vi "STD Cal Data.vi"(8 "error in":errorcluster caption="에러 입력(에러 없음)", 9 "Data in":string[][](array[string]), 10 "문자열":string, 11 "Func_ext":string) -> (0 "error out":errorcluster caption="에러 출력", 1 "Data Out":string[][](array[string]), 3 "Func_ext Out":string, 4 "Data Out 2":string[](array[string]), 6 "Cal STD":string[][](array[string]))   [LabVIEW 2020]
uses:
  Controls/Cmd_Var Data IO.ctl
  Controls/Cmd_File path.ctl
  Controls/Cmd_File Type.ctl
  Controls/Cmd_STD select.ctl
  <vilib>/Utility/file.llb/Read Delimited Spreadsheet (string).vi
  Public/Polymorph/Data Class_2D Str.vi
  Public/Polymorph/Array Dedup_1D Str.vi
  Public/Polymorph/Sort_2D Str.vi
  Variables/Global_Cal Info.vi
panel:
  out "Cal STD in":string[][](array[string])
  out "Condition Default":string[][](array[string])
  out "데이터오류?":bool
  out "생성오류?":bool
  out "Condition":string[][](array[string])
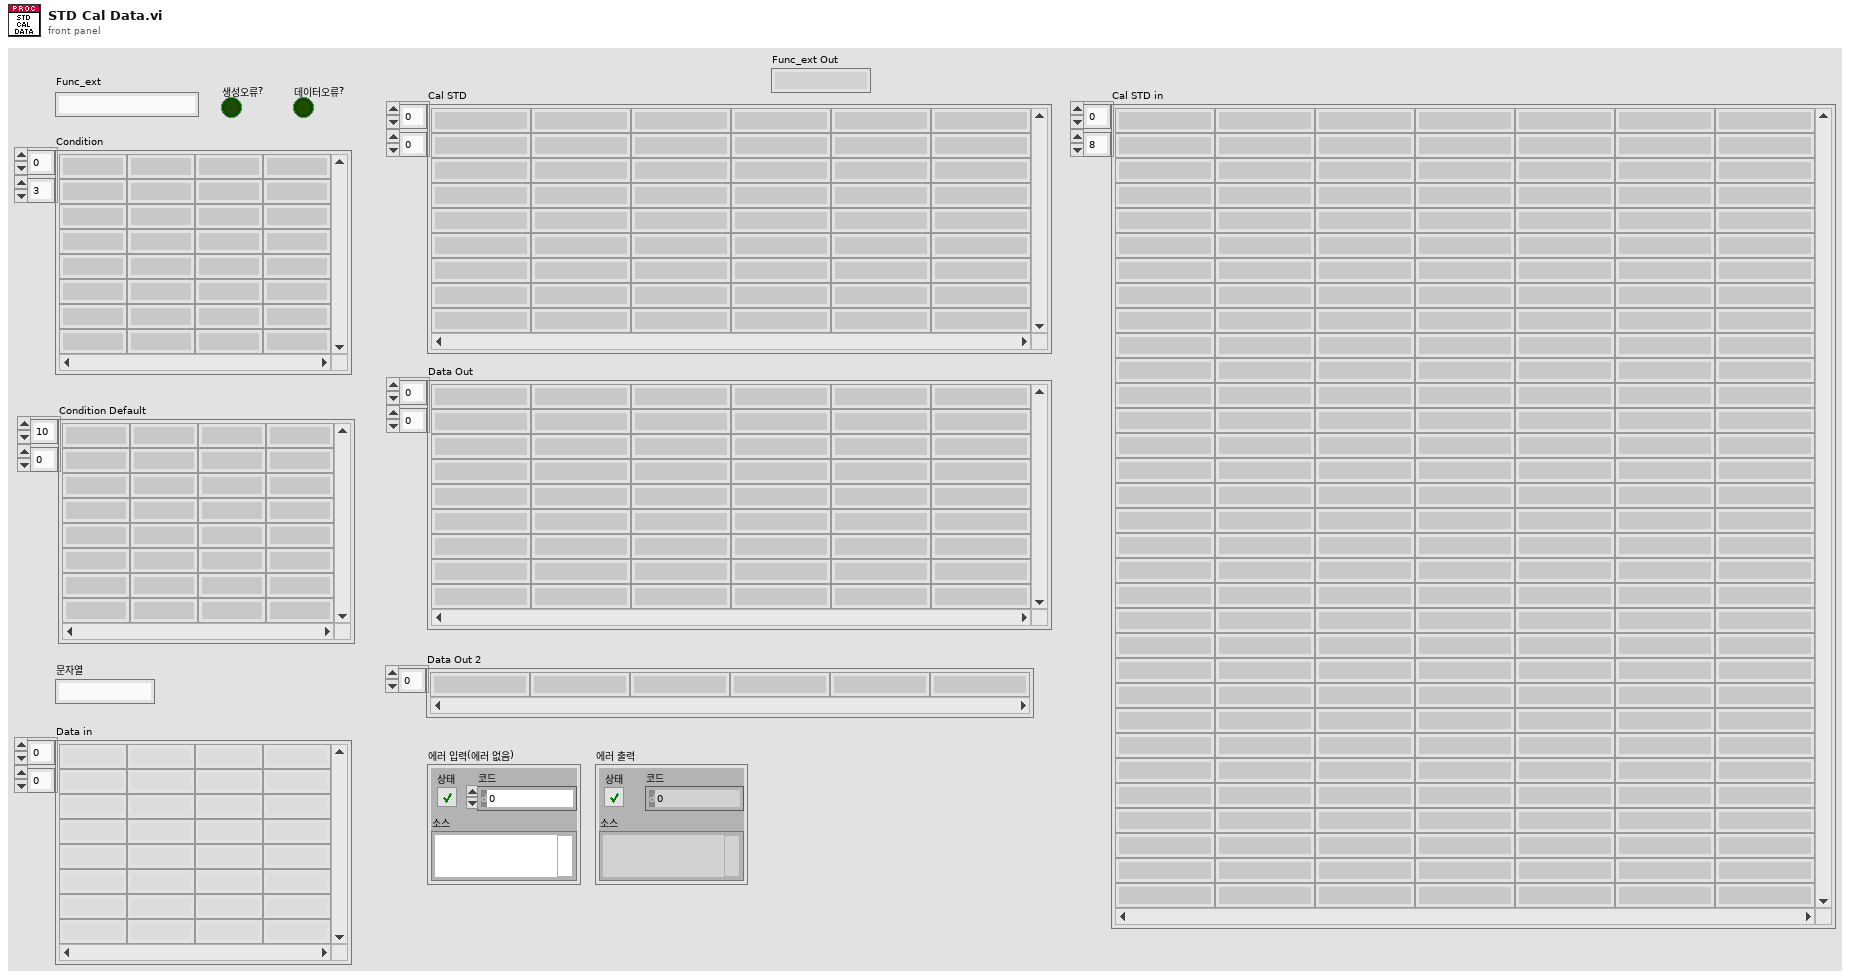
[diagram p1: front panel]
types:
  T1 = typedef "Cmd_Var Data IO.ctl" = enum16{"Condition", "Condition Default", "Condition_Temp", "Resolution", "Resolution Default", "Resolution Old", "Spec", "Spec Default", "Spec Old", "Spec Temp", "Result", "Result2", "Result3", "Result_Temp", "Result_ADJ", "Result_ADJ2", "STD1", "STD2", "STD3", "STD4", "STD5", "STD Temp", "CMC", "CMC Default"}
  T2 = typedef "Cmd_File Type.ctl" = enum16{"엑셀", "엑셀(2003)", "텍스트", "설정", "2진", "VI", "CSV", "LOG", "폴더"}
  T3 = typedef "Cmd_File path.ctl" = enum16{"에러로그", "데이터파일경로", "성적서원본", "지난성적서", "Data Files", "경로생성", "Updater", "Template", "설정파일경로", "FTP Upload", "Update 경로", "어플리케이션"}
  T4 = typedef "Cmd_STD select.ctl" = enum16{"기본", "DMM", "Electronic Micrometer", "Fine Angle Generator", "Measuring Projector", "Precision Square", "Power Supply", "Ring Gauge", "Straight Edge", "Thermo-Hygrometer", "Calibrator"}
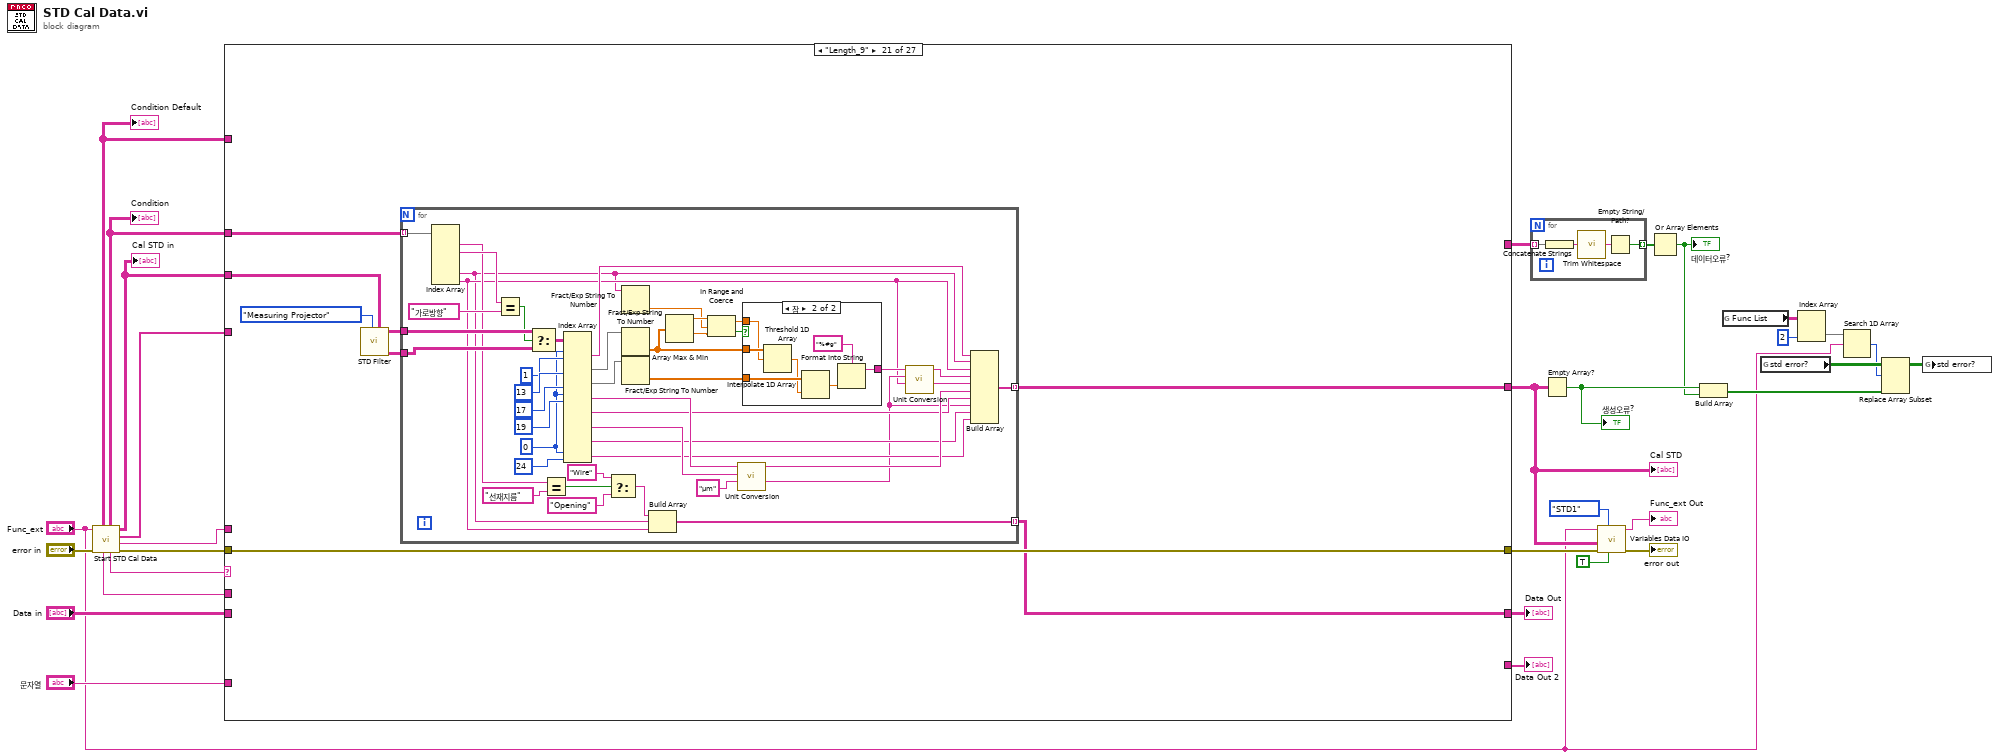
[diagram p0: block diagram]
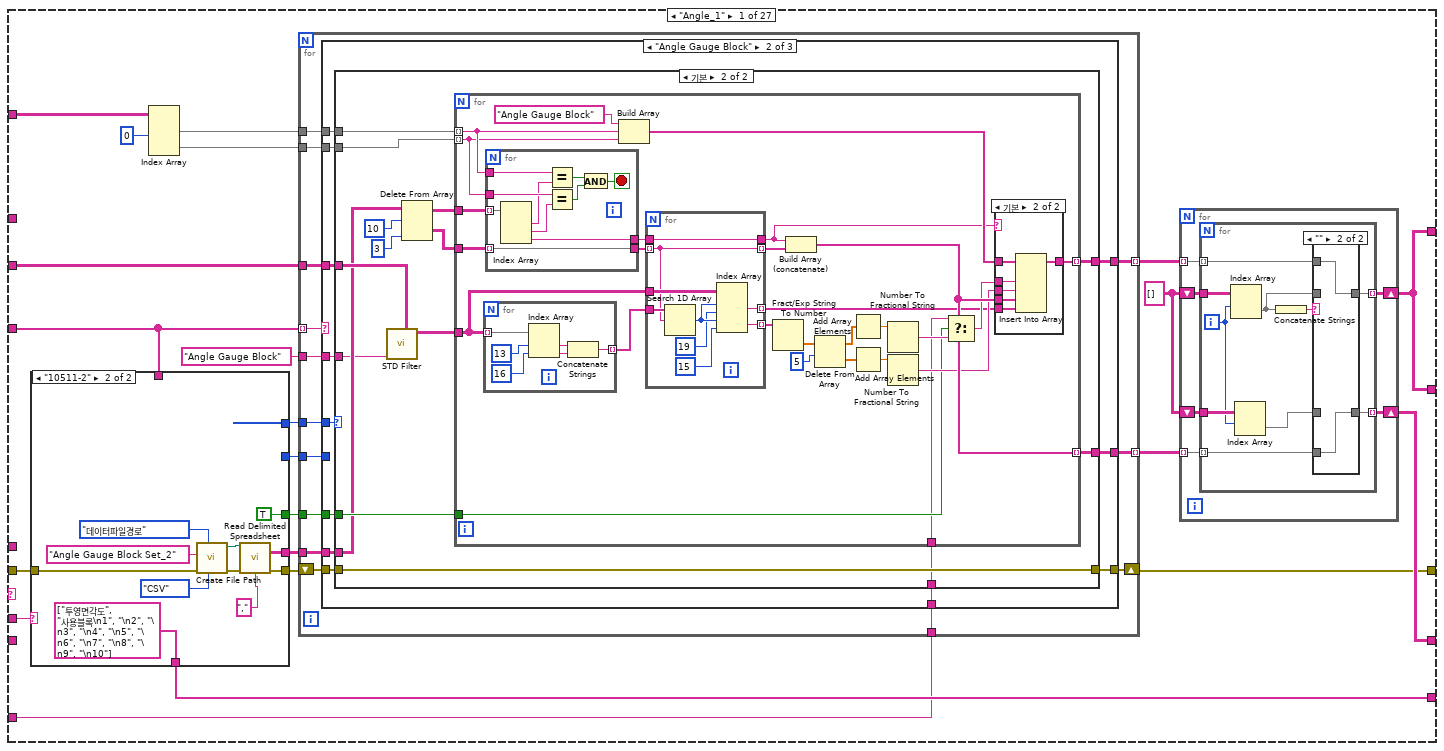
[diagram p2: hidden frame]
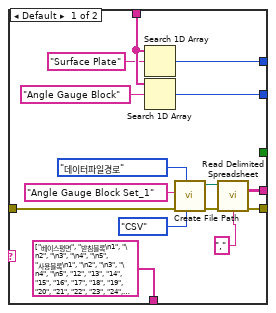
[diagram p3: hidden frame]
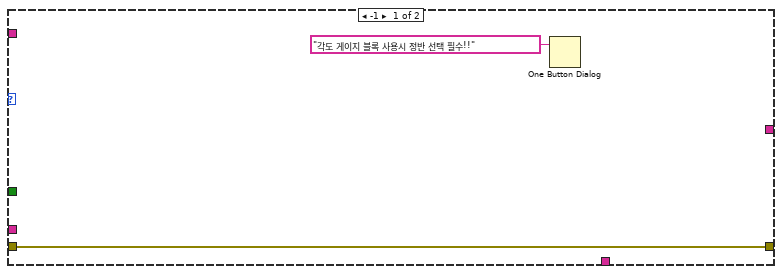
[diagram p6: hidden frame]
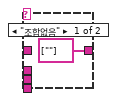
[diagram p7: hidden frame]
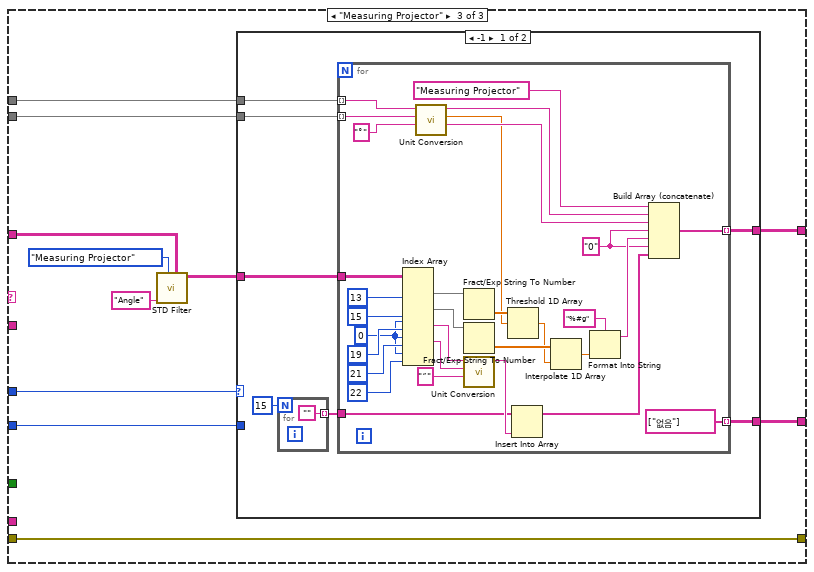
[diagram p8: hidden frame]
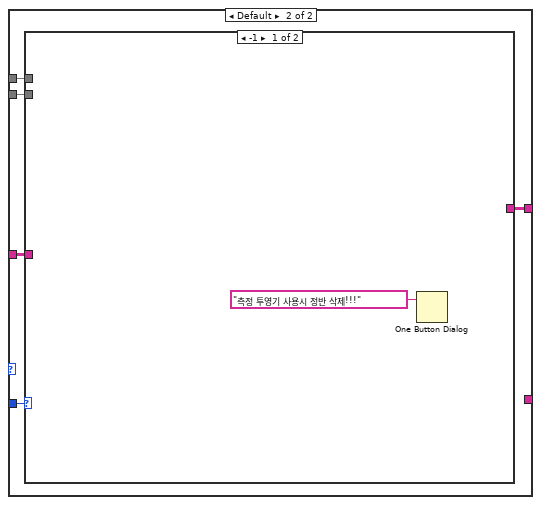
[diagram p9: hidden frame]
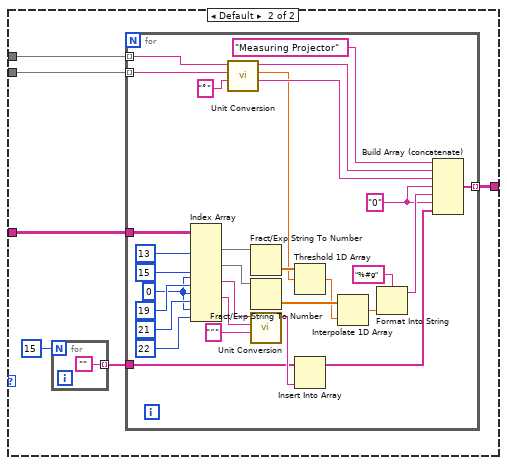
[diagram p10: hidden frame]
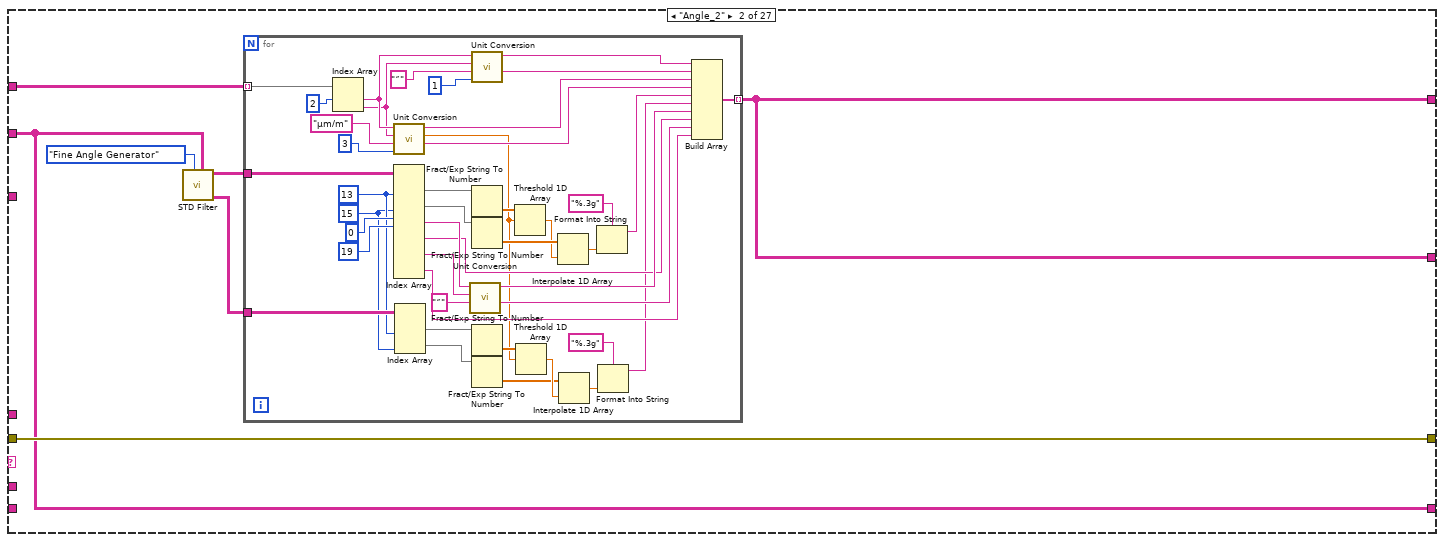
[diagram p11: hidden frame]
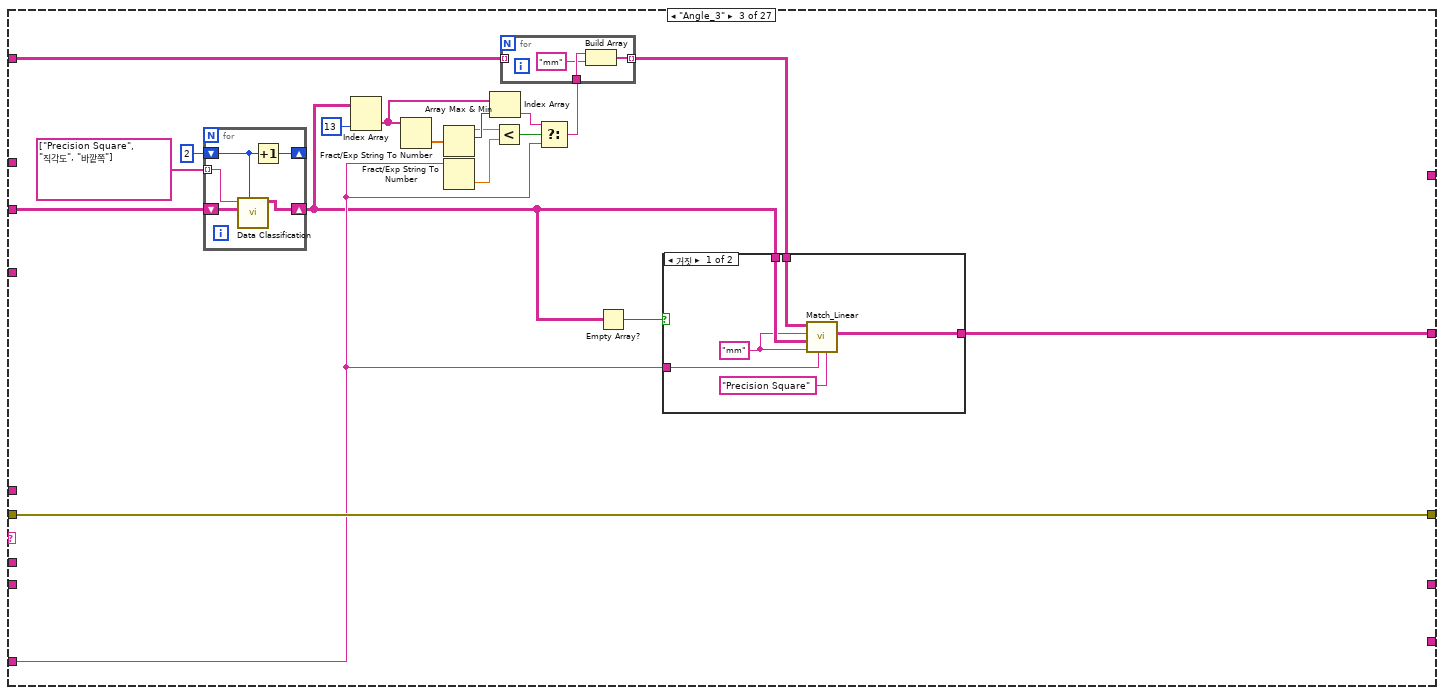
[diagram p12: hidden frame]
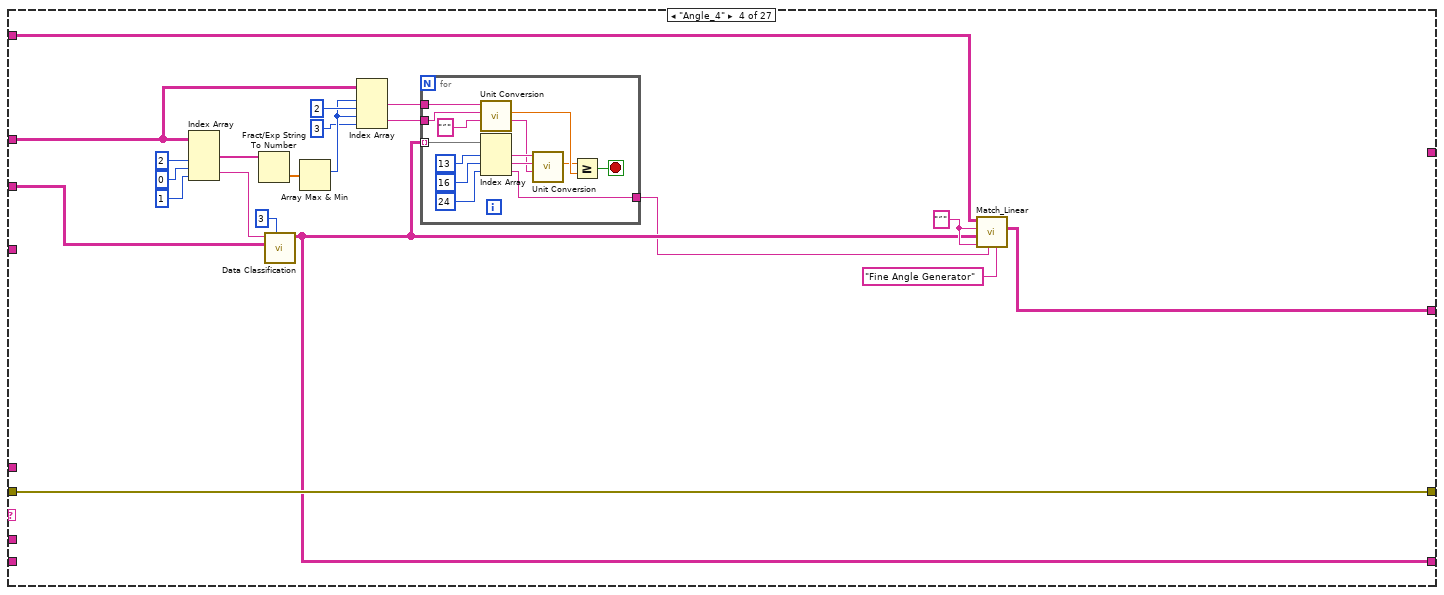
[diagram p14: hidden frame]
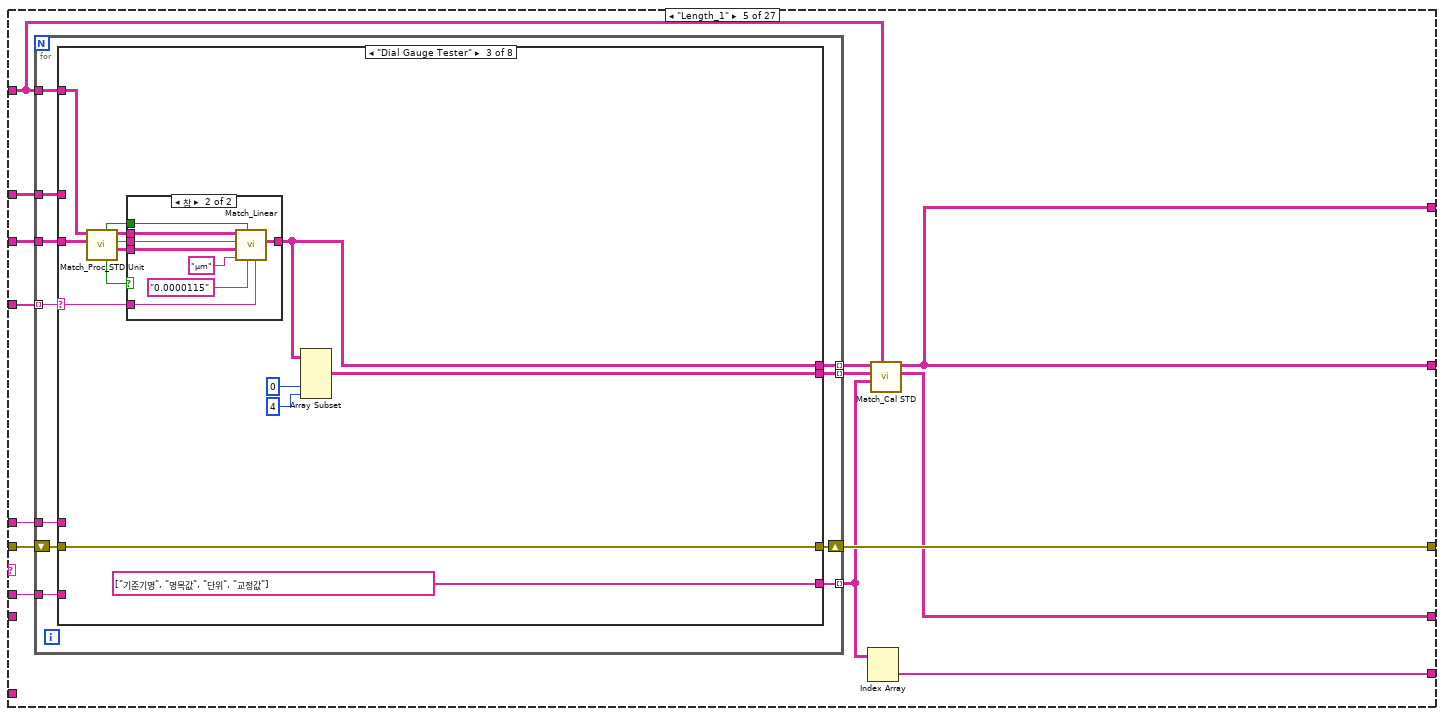
[diagram p15: hidden frame]
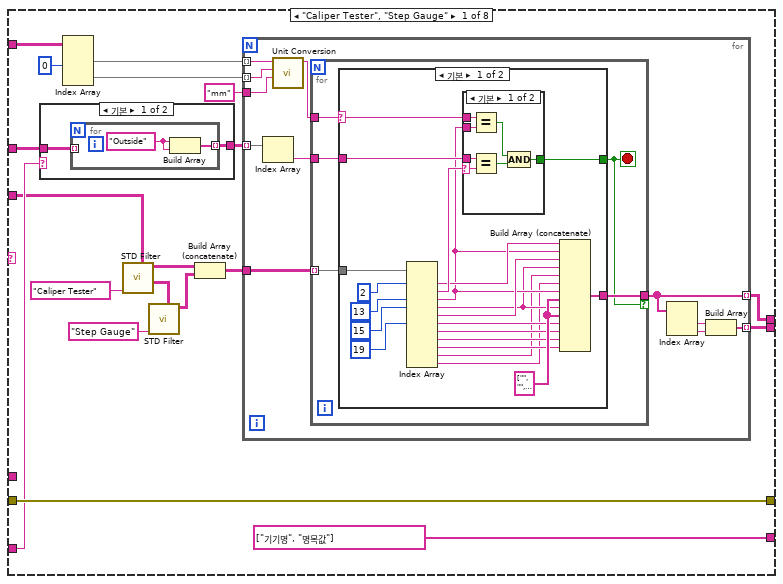
[diagram p16: hidden frame]
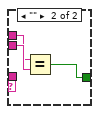
[diagram p17: hidden frame]
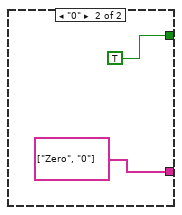
[diagram p18: hidden frame]
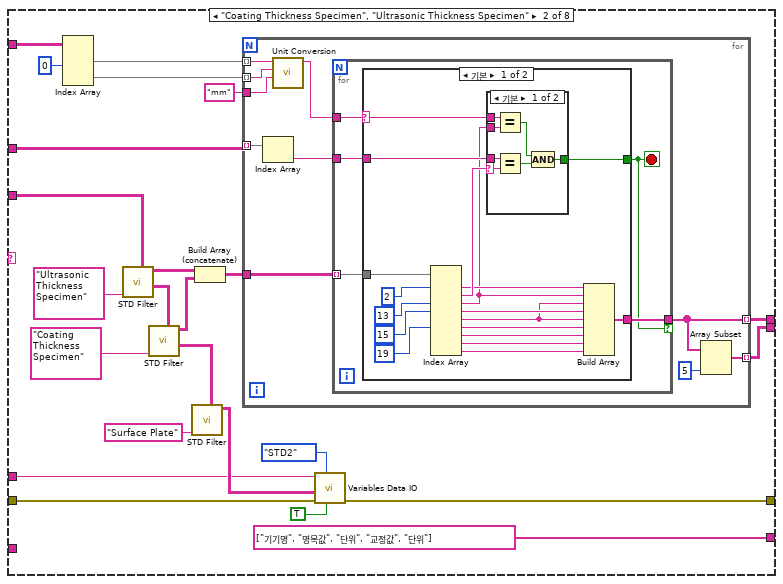
[diagram p20: hidden frame]
diagram:
  n1 = call "Start STD Cal Data.vi"("에러 입력"="error in", "Func_ext"="Func_ext") -> ("에러 출력"=w21:errorcluster, "Func_ext Out"=w5:string, "기준기명 out"=w3:string[], "Cal STD"=w4:string[][], "Func_ext_R제거"=w1:string, "Condition"=w6:string[][], "세부분류코드"=w2:string, "Condition Default"=w7:string[][])  [unwired: 2 in]
  "Condition" <- w6
  "Condition Default" <- w7
  "Cal STD in" <- w4
  n2 = case shown="\"Length_9\"" w1 {
    tunnel: w21 -> [w38 w299 w363 w398 w426 w757 w826 w898 w931 w980 w1054 w1071 w1094 w1106 w1244 w1285 w1607 w1627 w1657 w1788 w1820 w1887 w1921 w1974 w2027 w2044 w2075]
    tunnel: [w51 w299 w363 w398 w425 w756 w825 w897 w921 w961 w1054 w1071 w1093 w1106 w1241 w1286 w1607 w1627 w1656 w1780 w1820 w1887 w1921 w1969 w2023 w2044 w2075] -> w31
    tunnel: w4 -> [w53 w297 w362 w396 w421 w733 w828 w899 w917 w982 w1050 w1067 w1096 w1102 w1252 w1284 w1571 w1623 w1661 w1782 w1815 w1876 w1920 w1976 w2029 w2043 _]
    tunnel: [w50 w300 w347 w394 w419 w754 w837 w904 w908 w984 w1049 w1057 w1098 w1104 w1256 w1288 w1590 w1626 w1662 w1787 w1819 w1884 w1916 w1977 w2009 w2037 w2074] -> w23
    tunnel: [w52 w297 _ w388 w418 w752 w836 w903 w936 w967 _ w1072 w1099 w1103 _ w1282 w1572 w1621 w1659 w1781 w1817 _ w1905 w1972 w2009 w2035 _] -> w28
    tunnel: w6 -> [_ w301 _ w384 w422 w761 _ w895 _ w983 _ _ _ _ _ _ w1573 _ w1663 _ w1818 w1877 w1913 _ _ _ _]
    tunnel: [w50 w300 _ _ w419 w754 w837 w904 _ w984 w1049 _ w1098 w1104 w1256 w1288 w1590 w1626 w1662 w1787 _ _ w1916 w1977 w2009 w2037 w2074] -> w22
    tunnel: w7 -> [w33 _ w359 w387 w416 w749 w824 _ w914 w957 _ w1068 w1097 w1105 w1257 w1287 _ w1625 _ w1786 _ _ _ w1957 _ w2041 _]
    tunnel: w5 -> [_ _ _ _ w423 w759 w827 w900 w930 w978 _ _ w1092 _ w1245 w1280 _ _ w1655 w1779 _ _ _ w1973 w2026 _ _]
    tunnel: w2 -> [w43 _ _ _ w424 w758 _ w901 _ _ _ _ w1095 w1101 _ w1281 _ _ w1660 w1778 _ _ _ _ _ _ _]
    tunnel: [w42 _ _ _ w415 w750 _ w902 w929 w964 _ _ _ _ _ _ _ _ w1658 w1785 _ w1882 _ _ _ _ _] -> w11
    tunnel: "Data in" -> [_ _ _ _ _ w732 _ w896 _ _ w1053 _ _ w1100 _ _ _ _ _ w1784 _ _ _ _ _ _ _]
    tunnel: "문자열" -> [w40 _ w349 _ _ _ _ _ w913 w947 _ _ _ _ _ w1279 _ _ w1654 w1783 _ _ _ w1971 w2025 _ _]
    tunnel: w3 -> [w36 _ _ _ w414 w748 w823 _ _ _ _ _ _ _ _ _ _ _ _ _ _ _ _ _ _ _ _]
    frame "Angle_1" {
      w48 = string[][] []
      n3 = case shown="\"10511-2\"" w43 {
        tunnel: [w67 _] -> w49
        tunnel: w36 -> [w66 _]
        tunnel: [w65 _] -> w46
        tunnel: [string[] ["베이스평면", "받침블록\n1", "\n2", "\n3", "\n4", "\n5", "사용블록\n1", "\n2", "\n3", "\n4", "\n5", "12", "13", "14", "15", "16", "17", "18", "19", "20", "21", "22", "23", "24", "25", "26", "27", "28", "29", "30"] ("열 헤더 문자열[]") string[] ["투영면각도", "사용블록\n1", "\n2", "\n3", "\n4", "\n5", "\n6", "\n7", "\n8", "\n9", "\n10"] ("열 헤더 문자열[]")] -> w42
        tunnel: [_ TRUE] -> w41
        tunnel: [w60 w73] -> w39
        tunnel: w38 -> [w63 w77]
        tunnel: [w57 w69] -> w37
        frame Default {
          n4 = Search 1D Array(1D array=w66, element="Surface Plate" ("원소")) -> (index of element=w65:i32)  [unwired: 1 in]
          n5 = Search 1D Array(1D array=w66, element="Angle Gauge Block" ("검색 문자열")) -> (index of element=w67:i32)  [unwired: 1 in]
          n6 = call "Create File Path.vi"("파일타입"=Cmd_File_Type."CSV", "항목"=Cmd_File_path."데이터파일경로", "에러 입력"=w63, "문자열 in"="Angle Gauge Block Set_1") -> ("error out"=w60:errorcluster, "파일경로"=w56:path)  [unwired: 4 in, 2 out]
          n7 = call-poly <vilib>:"Read Delimited Spreadsheet.vi"("file path (dialog if empty)"=w56, "error in (no error)"=w60, "delimiter (\\t)"="," ("delimiter (\\t)")) -> ("all rows"=w57:string[][])  [unwired: 7 in, 5 out]
        }
        frame "10511-2" {
          n8 = call "Create File Path.vi"("파일타입"=Cmd_File_Type."CSV", "항목"=Cmd_File_path."데이터파일경로", "에러 입력"=w77, "문자열 in"="Angle Gauge Block Set_2") -> ("error out"=w74:errorcluster, "파일경로"=w75:path)  [unwired: 4 in, 2 out]
          n9 = call-poly <vilib>:"Read Delimited Spreadsheet.vi"("file path (dialog if empty)"=w75, "error in (no error)"=w74, "delimiter (\\t)"="," ("delimiter (\\t)")) -> ("all rows"=w69:string[][], "error out"=w73:errorcluster)  [unwired: 7 in, 4 out]
        }
      }
      n10 = Index Array(array=w33, index (col) #1=0 ("비활성화된 인덱스 (열)")) -> (element #1=w32:string[], element #2=w45:string[])  [unwired: 3 in]
      n11 = for {
        tunnel: w32 -> [w110]
        tunnel: w45 -> [w109]
        tunnel: [w108] -> w47 mode=indexing
        tunnel: [w107] -> w34 mode=indexing
        tunnel: w53 -> [w106]
        tunnel: w36 -> [w105] mode=indexing
        shift-right: [w111] -> w51
        shift-left: w39 -> [w112]
        tunnel: w46 -> [w104]
        tunnel: w49 -> [w103]
        tunnel: w41 -> [w102]
        tunnel: w40 -> [w101]
        tunnel: w37 -> [w100]
        tunnel: "Angle Gauge Block" ("검색 문자열") -> [w99]
        n12 = case shown="\"Angle Gauge Block\"" w105 {
          tunnel: w112 -> [w113 w122 w207]
          tunnel: w106 -> [_ w123 w204]
          tunnel: [w113 w121 w207] -> w111
          tunnel: w110 -> [_ w125 w212]
          tunnel: w109 -> [_ w124 w211]
          tunnel: [_ w120 w206] -> w108
          tunnel: [_ w119 w210] -> w107
          tunnel: w104 -> [_ w118 w209]
          tunnel: w103 -> [_ _ w208]
          tunnel: w102 -> [_ w117 _]
          tunnel: w101 -> [_ w116 _]
          tunnel: w100 -> [_ w115 _]
          tunnel: w99 -> [_ w114 _]
          frame Default {
          }
          frame "Angle Gauge Block" {
            n13 = case shown="기본" w118 {
              tunnel: w125 -> [_ w129]
              tunnel: w124 -> [_ w131]
              tunnel: w123 -> [_ w133]
              tunnel: w122 -> [w127 w136]
              tunnel: [w127 w136] -> w121
              tunnel: [_ w138] -> w120
              tunnel: [_ w137] -> w119
              tunnel: w117 -> [_ w135]
              tunnel: w116 -> [_ w134]
              tunnel: w115 -> [_ w130]
              tunnel: w114 -> [_ w128]
              frame -1 {
                n14 = One Button Dialog(message="각도 게이지 블록 사용시 정반 선택 필수!!" ("메시지")) -> ()  [unwired: 1 in, 1 out]
              }
              frame Default {
                n15 = call "STD Filter.vi"("Cal STD in"=w133, "문자열(option, STD)"=w128) -> ("DATA 출력"=w132:string[][])  [unwired: 5 in, 4 out]
                n16 = Delete From Array(array=w130, length=10 ("길이"), index (col)=3 ("비활성화된 인덱스 (열)")) -> (deleted portion=w140:string[][], array with subset deleted=w139:string[][])  [unwired: 1 in]
                n17 = for {
                  tunnel: w140 -> [w168]
                  tunnel: w132 -> [w143]
                  tunnel: w129 -> [w145] mode=indexing
                  tunnel: w131 -> [w144] mode=indexing
                  tunnel: [w165] -> w138 mode=indexing
                  tunnel: w139 -> [w169]
                  tunnel: [w164] -> w137 mode=indexing
                  tunnel: w135 -> [w154]
                  tunnel: w134 -> [w153]
                  n18 = for {
                    tunnel: w143 -> [w171] mode=indexing
                    tunnel: [w170] -> w150 mode=indexing
                    n19 = Index Array(array=w171, index #1=13 ("인덱스"), index #2=16 ("인덱스")) -> (element #1=w173:string, element #2=w172:string)
                    n20 = Concatenate Strings(w173, w172) -> (w170:string)
                  }
                  n21 = for {
                    tunnel: w169 -> [w194] mode=indexing
                    tunnel: w145 -> [w196]
                    tunnel: w144 -> [w195]
                    tunnel: w168 -> [w197] mode=indexing
                    tunnel: [w197] -> w163
                    tunnel: [w198] -> w147
                    stop <- w199 stop-if-true
                    n22 = Index Array(array=w194) -> (element #1=w193:string, element #2=w192:string, element #3=w198:string)  [unwired: 3 in]
                    n23 = Equal?(x=w196, y=w193) -> (x = y?=w201:bool)
                    n24 = Equal?(x=w195, y=w192) -> (x = y?=w200:bool)
                    n25 = And(x=w201, y=w200) -> (x .and. y?=w199:bool)
                  }
                  n26 = Build Array("Angle Gauge Block" ("검색 문자열"), w145, w144) -> (w166:string[])
                  n27 = for {
                    tunnel: w150 -> [w189]
                    tunnel: w143 -> [w191]
                    tunnel: w163 -> [w184] mode=indexing
                    tunnel: [w188] -> w152 mode=indexing
                    tunnel: [w185] -> w149 mode=indexing
                    tunnel: [w184] -> w148 mode=indexing
                    tunnel: w147 -> [w183]
                    tunnel: [w183] -> w146
                    n28 = Search 1D Array(1D array=w189, element=w184) -> (index of element=w187:i32)  [unwired: 1 in]
                    n29 = Index Array(array=w191, index (row) #1=w187, index (col) #1=19 ("인덱스 (열)"), index (row) #2=w187, index (col) #2=15 ("비활성화된 인덱스 (열)")) -> (element #1=w185:string, element #2=w188:string)
                  }
                  n30 = Fract/Exp String To Number(string=w152) -> (number=w151:dbl[])  [unwired: 3 in, 1 out]
                  n31 = Build Array (concatenate)(w146, w148) -> (w165:string[])
                  n32 = Delete From Array(array=w151, length=5 ("길이")) -> (deleted portion=w160:dbl[], array with subset deleted=w161:dbl[])  [unwired: 1 in]
                  n33 = Add Array Elements(numeric array=w161) -> (sum=w159:dbl)
                  n34 = Add Array Elements(numeric array=w160) -> (sum=w158:dbl)
                  n35 = Number To Fractional String(number=w159) -> (F-format string=w156:string)  [unwired: 3 in]
                  n36 = Number To Fractional String(number=w158) -> (F-format string=w157:string)  [unwired: 3 in]
                  n37 = Select(t=w153, s=w154, f=w156) -> (s? t:f=w155:string)
                  n38 = case shown="기본" w146 {
                    tunnel: w166 -> [_ w182]
                    tunnel: w165 -> [_ w181]
                    tunnel: [string[] [""] w180] -> w164
                    tunnel: w155 -> [_ w179]
                    tunnel: w157 -> [_ w178]
                    tunnel: w149 -> [_ w177]
                    frame "조합없음" {
                    }
                    frame Default {
                      n39 = Insert Into Array(array=w182, new element #1=w179, new element #2=w178, new element #3=w181, new element #4=w177) -> (w180:string[])  [unwired: 1 in]
                    }
                  }
                }
              }
            }
          }
          frame "Measuring Projector" {
            n40 = call "STD Filter.vi"("Cal STD in"=w204, "STD select"=Cmd_STD_select."Measuring Projector", "문자열(option, STD)"="Angle" ("검색 문자열")) -> ("DATA 출력"=w202:string[][])  [unwired: 4 in, 4 out]
            n41 = case shown="-1" w209 {
              tunnel: w212 -> [w219 w256]
              tunnel: w211 -> [w218 w255]
              tunnel: [w217 w254] -> w210
              tunnel: [w216 _] -> w206
              tunnel: w208 -> [_ w253]
              tunnel: w202 -> [w213 w252]
              frame -1 {
                n42 = for {
                  N: 15 -> [_]
                  tunnel: [""] -> w214 mode=indexing
                }
                n43 = for {
                  tunnel: w213 -> [w251]
                  tunnel: w219 -> [w245] mode=indexing
                  tunnel: w218 -> [w244] mode=indexing
                  tunnel: [w242] -> w217 mode=indexing
                  tunnel: [string[] ["없음"]] -> w216 mode=indexing
                  tunnel: w214 -> [w221]
                  w224 = "0" ("원소")
                  w229 = 0 ("인덱스 (열)")
                  n44 = Index Array(array=w251, index (col) #1=13 ("인덱스 (행)"), index (col) #2=15 ("인덱스 (행)"), index (row) #3=w229, index (col) #3=19 ("인덱스 (열)"), index (row) #4=w229, index (col) #4=21 ("인덱스 (열)"), index (row) #5=w229, index (col) #5=22 ("인덱스 (열)")) -> (element #1=w239:string[], element #2=w250:string[], element #3=w233:string, element #4=w228:string)  [unwired: 2 in, 1 out]
                  n45 = call "Unit Conversion.vi"("환산단위"="˚", "입력단위"=w244, "입력값"=w245) -> ("환산단위"=w240:string, "환산값 (DBL)"=w231:dbl, "환산값 (string)"=w241:string)  [unwired: 3 in, 3 out]
                  n46 = Fract/Exp String To Number(string=w239) -> (number=w238:dbl[])  [unwired: 3 in, 1 out]
                  n47 = Fract/Exp String To Number(string=w250) -> (number=w249:dbl[])  [unwired: 3 in, 1 out]
                  n48 = call "Unit Conversion.vi"("환산단위"="˝", "입력단위"=w228, "입력값"=w233) -> ("환산값 (string)"=w223:string)  [unwired: 3 in, 5 out]
                  n49 = Threshold 1D Array(2:w231, 3:w238) -> (0:w232:dbl)  [unwired: 1 in]
                  n50 = Insert Into Array(array=w221, new element=w223) -> (w222:string[])  [unwired: 1 in]
                  n51 = Interpolate 1D Array(1:w232, 2:w249) -> (0:w246:dbl)
                  n52 = Format Into String(format string="%#g" ("포맷 문자열"), w246) -> (resulting string=w225:string)  [unwired: 2 in, 1 out]
                  n53 = Build Array (concatenate)("Measuring Projector" ("검색 문자열"), w241, w240, w224, w225, w224, w222) -> (w242:string[])
                }
              }
              frame Default {
                n54 = case shown="-1" w253 {
                  tunnel: w256 -> [_ w263]
                  tunnel: w255 -> [_ w262]
                  tunnel: [_ w261] -> w254
                  tunnel: w252 -> [_ w258]
                  frame -1 {
                    n55 = One Button Dialog(message="측정 투영기 사용시 정반 삭제!!!" ("메시지")) -> ()  [unwired: 1 in, 1 out]
                  }
                  frame Default {
                    n56 = for {
                      N: 15 -> [_]
                      tunnel: [""] -> w259 mode=indexing
                    }
                    n57 = for {
                      tunnel: w258 -> [w294]
                      tunnel: w263 -> [w288] mode=indexing
                      tunnel: w262 -> [w287] mode=indexing
                      tunnel: [w285] -> w261 mode=indexing
                      tunnel: w259 -> [w265]
                      w268 = "0" ("원소")
                      w272 = 0 ("인덱스 (열)")
                      n58 = Index Array(array=w294, index (col) #1=13 ("인덱스 (행)"), index (col) #2=15 ("인덱스 (행)"), index (row) #3=w272, index (col) #3=19 ("인덱스 (열)"), index (row) #4=w272, index (col) #4=21 ("인덱스 (열)"), index (row) #5=w272, index (col) #5=22 ("인덱스 (열)")) -> (element #1=w282:string[], element #2=w293:string[], element #3=w276:string, element #4=w271:string)  [unwired: 2 in, 1 out]
                      n59 = call "Unit Conversion.vi"("환산단위"="˚", "입력단위"=w287, "입력값"=w288) -> ("환산단위"=w283:string, "환산값 (DBL)"=w274:dbl, "환산값 (string)"=w284:string)  [unwired: 3 in, 3 out]
                      n60 = Fract/Exp String To Number(string=w282) -> (number=w281:dbl[])  [unwired: 3 in, 1 out]
                      n61 = Fract/Exp String To Number(string=w293) -> (number=w292:dbl[])  [unwired: 3 in, 1 out]
                      n62 = call "Unit Conversion.vi"("환산단위"="˝", "입력단위"=w271, "입력값"=w276) -> ("환산값 (string)"=w267:string)  [unwired: 3 in, 5 out]
                      n63 = Threshold 1D Array(2:w274, 3:w281) -> (0:w275:dbl)  [unwired: 1 in]
                      n64 = Insert Into Array(array=w265, new element=w267) -> (w266:string[])  [unwired: 1 in]
                      n65 = Interpolate 1D Array(1:w275, 2:w292) -> (0:w289:dbl)
                      n66 = Format Into String(format string="%#g" ("포맷 문자열"), w289) -> (resulting string=w269:string)  [unwired: 2 in, 1 out]
                      n67 = Build Array (concatenate)("Measuring Projector" ("검색 문자열"), w284, w283, w268, w269, w268, w266) -> (w285:string[])
                    }
                  }
                }
              }
            }
          }
        }
      }
      n68 = for {
        tunnel: w34 -> [w84] mode=indexing
        tunnel: w47 -> [w81] mode=indexing
        shift-right: [w83] -> w50
        shift-left: w48 -> [w82]
        shift-right: [w79] -> w52
        shift-left: w48 -> [w80]
        n69 = for {
          tunnel: w84 -> [w93] mode=indexing
          tunnel: [w92] -> w83 mode=indexing
          tunnel: w82 -> [w91]
          tunnel: w81 -> [w89] mode=indexing
          tunnel: w80 -> [w88]
          tunnel: [w85] -> w79 mode=indexing
          i -> [w87]
          n70 = Index Array(array=w91, index (row)=w87) -> (element=w90:string[])  [unwired: 1 in]
          n71 = Index Array(array=w88, index (row)=w87) -> (element=w86:string[])  [unwired: 1 in]
          n72 = Concatenate Strings(w90) -> (w94:string)
          n73 = case shown="\"\"" w94 {
            tunnel: w93 -> [_ w98]
            tunnel: [w96 w98] -> w92
            tunnel: w90 -> [w96 _]
            tunnel: [w95 w97] -> w85
            tunnel: w89 -> [_ w97]
            tunnel: w86 -> [w95 _]
            frame Default {
            }
            frame "" {
            }
          }
        }
      }
    }
    frame "Angle_2" {
      n74 = call "STD Filter.vi"("Cal STD in"=w297, "STD select"=Cmd_STD_select."Fine Angle Generator") -> ("제외 DATA 출력"=w295:string[][], "DATA 출력"=w296:string[][])  [unwired: 5 in, 3 out]
      n75 = for {
        tunnel: w301 -> [w344] mode=indexing
        tunnel: w296 -> [w341]
        tunnel: [w339] -> w300 mode=indexing
        tunnel: w295 -> [w314]
        w310 = 15 ("인덱스 (행)")
        w311 = 13 ("인덱스 (행)")
        n76 = Index Array(array=w344, index #1=2 ("인덱스")) -> (element #1=w307:string, element #2=w306:string)  [unwired: 1 in]
        n77 = call "Unit Conversion.vi"("소수점 자리수"=3, "환산단위"="μm/m", "입력단위"=w306, "입력값"=w307) -> ("환산단위"=w326:string, "환산값 (DBL)"=w313:dbl, "환산값 (string)"=w340:string)  [unwired: 2 in, 3 out]
        n78 = Index Array(array=w341, index (col) #1=w311, index (col) #2=w310, index (row) #3=0 ("인덱스 (열)"), index (col) #3=19 ("인덱스 (열)")) -> (element #1=w334:string[], element #2=w338:string[], element #3=w331:string, element #4=w322:string, element #5=w323:string, element #6=w324:string)  [unwired: 8 in]
        n79 = Index Array(array=w314, index (col) #1=w311, index (col) #2=w310) -> (element #1=w318:string[], element #2=w315:string[])  [unwired: 2 in]
        n80 = call "Unit Conversion.vi"("환산단위"="˝", "입력단위"=w323, "입력값"=w331) -> ("환산단위"=w327:string, "환산값 (string)"=w328:string)  [unwired: 3 in, 4 out]
        n81 = call "Unit Conversion.vi"("소수점 자리수"=1, "환산단위"="˝", "입력단위"=w306, "입력값"=w307) -> ("환산단위"=w303:string, "환산값 (string)"=w304:string)  [unwired: 2 in, 4 out]
        n82 = Fract/Exp String To Number(string=w334) -> (number=w333:dbl[])  [unwired: 3 in, 1 out]
        n83 = Fract/Exp String To Number(string=w338) -> (number=w337:dbl[])  [unwired: 3 in, 1 out]
        n84 = Fract/Exp String To Number(string=w318) -> (number=w319:dbl[])  [unwired: 3 in, 1 out]
        n85 = Fract/Exp String To Number(string=w315) -> (number=w316:dbl[])  [unwired: 3 in, 1 out]
        n86 = Threshold 1D Array(2:w313, 3:w333) -> (0:w330:dbl)  [unwired: 1 in]
        n87 = Threshold 1D Array(2:w313, 3:w319) -> (0:w320:dbl)  [unwired: 1 in]
        n88 = Interpolate 1D Array(1:w330, 2:w337) -> (0:w336:dbl)
        n89 = Interpolate 1D Array(1:w320, 2:w316) -> (0:w317:dbl)
        n90 = Format Into String(format string="%.3g" ("포맷 문자열"), w336) -> (resulting string=w335:string)  [unwired: 2 in, 1 out]
        n91 = Format Into String(format string="%.3g" ("포맷 문자열"), w317) -> (resulting string=w312:string)  [unwired: 2 in, 1 out]
        n92 = Build Array(w304, w303, w340, w326, w335, w312, w328, w322, w327, w324) -> (w339:string[])
      }
    }
    frame "Angle_3" {
      n93 = for {
        tunnel: string[] ["Precision Square", "직각도", "바깥쪽"] -> [w375] mode=indexing
        shift-right: [w373] -> _
        shift-left: 2 ("인덱스") -> [w374]
        shift-right: [w376] -> w346
        shift-left: w362 -> [w377]
        n94 = call-poly "Data Classification.vi"("인덱스"=w374, "DATA 입력"=w377, "검색 문자열"=w375) -> ("DATA 출력"=w376:string[][])  [unwired: 4 in, 4 out]
        n95 = Increment(x=w374) -> (x+1=w373:i32)
      }
      n96 = Index Array(array=w346, index (col)=13 ("비활성화된 인덱스 (열)")) -> (element=w355:string[])  [unwired: 1 in]
      n97 = Fract/Exp String To Number(string=w355) -> (number=w357:dbl[])  [unwired: 3 in, 1 out]
      n98 = Array Max & Min(array=w357) -> (max value=w354:dbl, max index (indices)=w356:i32)  [unwired: 2 out]
      n99 = Fract/Exp String To Number(string=w349) -> (number=w353:dbl)  [unwired: 3 in, 1 out]
      n100 = Index Array(array=w355, index=w356) -> (element=w351:string)
      n101 = Less?(x=w354, y=w353) -> (x < y?=w352:bool)
      n102 = Select(t=w351, s=w352, f=w349) -> (s? t:f=w350:string)
      n103 = for {
        tunnel: w359 -> [_] mode=indexing
        tunnel: w350 -> [w372]
        tunnel: [w370] -> w348 mode=indexing
        n104 = Build Array(w372, "mm" ("환산단위1")) -> (w370:string[])
      }
      n105 = Empty Array?(array=w346) -> (empty?=w345:bool)
      n106 = case shown="거짓" w345 {
        tunnel: w349 -> [w368 _]
        tunnel: w346 -> [w367 _]
        tunnel: w348 -> [w365 _]
        tunnel: [w364 _] -> w347
        frame False {
          w366 = "mm" ("환산단위1")
          n107 = call "Match_Linear.vi"("기준기명"="Precision Square", "열팽창계수(etc)"=w368, "환산단위(불확도)"=w366, "Cal STD in"=w367, "환산단위(교정값)"=w366, "Condition Default"=w365) -> ("Data out"=w364:string[][])  [unwired: 4 in, 1 out]
        }
        frame True {
        }
      }
    }
    frame "Angle_4" {
      w390 = "˝"
      n108 = Index Array(array=w384, index (col) #1=2 ("비활성화된 인덱스 (열)"), index (row) #2=0 ("인덱스 (행)"), index (col) #2=1 ("비활성화된 인덱스 (열)")) -> (element #1=w386:string[], element #2=w391:string)  [unwired: 1 in]
      n109 = Fract/Exp String To Number(string=w386) -> (number=w385:dbl[])  [unwired: 3 in, 1 out]
      n110 = call-poly "Data Classification.vi"("인덱스"=3, "DATA 입력"=w396, "검색 문자열"=w391) -> ("DATA 출력"=w388:string[][])  [unwired: 4 in, 4 out]
      n111 = Array Max & Min(array=w385) -> (max index (indices)=w382:i32)  [unwired: 3 out]
      n112 = Index Array(array=w384, index (row) #1=w382, index (col) #1=2 ("비활성화된 인덱스 (열)"), index (row) #2=w382, index (col) #2=3 ("비활성화된 인덱스 (열)")) -> (element #1=w380:string, element #2=w379:string)
      n113 = for {
        tunnel: w388 -> [w412] mode=indexing
        tunnel: w380 -> [w407]
        tunnel: w379 -> [w406]
        tunnel: [w400] -> w378
        stop <- w402 stop-if-true
        n114 = call "Unit Conversion.vi"("환산단위"="˝", "입력단위"=w406, "입력값"=w407) -> ("환산단위"=w399:string, "환산값 (DBL)"=w404:dbl)  [unwired: 3 in, 4 out]
        n115 = Index Array(array=w412, index #1=13 ("인덱스"), index #2=16 ("인덱스"), index #3=24 ("인덱스")) -> (element #1=w409:string, element #2=w408:string, element #3=w400:string)
        n116 = call "Unit Conversion.vi"("환산단위"=w399, "입력단위"=w408, "입력값"=w409) -> ("환산값 (DBL)"=w403:dbl)  [unwired: 3 in, 5 out]
        n117 = Greater Or Equal?(x=w403, y=w404) -> (x >= y?=w402:bool)
      }
      n118 = call "Match_Linear.vi"("기준기명"="Fine Angle Generator", "열팽창계수(etc)"=w378, "환산단위(불확도)"=w390, "Cal STD in"=w388, "환산단위(교정값)"=w390, "Condition Default"=w387) -> ("Data out"=w394:string[][])  [unwired: 4 in, 1 out]
    }
    frame "Length_1" {
      n119 = for {
        tunnel: [w436] -> w417 mode=indexing
        tunnel: [w434] -> w420 mode=indexing
        tunnel: w424 -> [w433]
        tunnel: [w432] -> w413 mode=indexing
        tunnel: w421 -> [w431]
        tunnel: w423 -> [w430]
        tunnel: w416 -> [w429]
        tunnel: w422 -> [w428]
        shift-right: [w435] -> w425
        shift-left: w426 -> [w437]
        tunnel: w414 -> [w427] mode=indexing
        n120 = case shown="\"Dial Gauge Tester\"" w427 {
          selector: w427 -> [_ _ w588 w606 _ w646 w668 _]
          tunnel: w437 -> [w456 w514 w593 w603 w637 w650 w660 w717]
          tunnel: w431 -> [w443 w525 w589 w607 w630 w645 w665 _]
          tunnel: [w453 w532 w590 w604 w635 w648 w669 _] -> w436
          tunnel: [w456 w513 w593 w603 w633 w650 w661 w717] -> w435
          tunnel: [w454 w533 w591 w605 w636 w649 w670 _] -> w434
          tunnel: w433 -> [w452 _ _ _ w632 _ w663 _]
          tunnel: [string[] ["기기명", "명목값"] string[] ["기기명", "명목값", "단위", "교정값", "단위"] string[] ["기준기명", "명목값", "단위", "교정값"] _ w634 string[] ["기준기명", "명목값", "단위", "교정값"] w662 _] -> w432
          tunnel: w430 -> [_ w512 _ _ w629 _ w659 _]
          tunnel: w429 -> [w447 w529 w585 w604 w631 w642 w664 _]
          tunnel: w428 -> [w451 w520 _ _ _ _ _ _]
          frame "Caliper Tester", "Step Gauge" {
            n121 = case shown="기본" w452 {
              tunnel: w451 -> [w507 w510]
              tunnel: [w506 w510] -> w450
              frame Default {
                n122 = for {
                  tunnel: [w509] -> w506 mode=indexing
                  tunnel: w507 -> [_] mode=indexing
                  w508 = "Outside" ("환산단위")
                  n123 = Build Array(w508, w508) -> (w509:string[])
                }
              }
              frame "10601-1" {
              }
            }
            n124 = Index Array(array=w447, index (col) #1=0 ("비활성화된 인덱스 (열)")) -> (element #1=w445:string[], element #2=w444:string[])  [unwired: 3 in]
            n125 = call "STD Filter.vi"("Cal STD in"=w443, "문자열(option, STD)"="Caliper Tester" ("검색 문자열")) -> ("Cal STD out"=w440:string[][], "DATA 출력"=w442:string[][])  [unwired: 5 in, 3 out]
            n126 = call "STD Filter.vi"("Cal STD in"=w440, "문자열(option, STD)"="Step Gauge" ("검색 문자열")) -> ("DATA 출력"=w441:string[][])  [unwired: 5 in, 4 out]
            n127 = Build Array (concatenate)(w442, w441) -> (w448:string[][])
            n128 = for {
              tunnel: w450 -> [w458] mode=indexing
              tunnel: w445 -> [w460] mode=indexing
              tunnel: w444 -> [w466] mode=indexing
              tunnel: "mm" ("환산단위") -> [w467]
              tunnel: [w463] -> w454 mode=indexing
              tunnel: w448 -> [w461]
              tunnel: [w462] -> w453 mode=indexing
              n129 = Index Array(array=w458) -> (element=w457:string)  [unwired: 1 in]
              n130 = call "Unit Conversion.vi"("환산단위"=w467, "입력단위"=w466, "입력값"=w460) -> ("환산값 (string)"=w459:string)  [unwired: 3 in, 5 out]
              n131 = for {
                tunnel: w461 -> [w471] mode=indexing
                tunnel: w457 -> [w472]
                tunnel: w459 -> [w468]
                tunnel: [w470] -> w463 if=w469
                stop <- w469 stop-if-true
                n132 = case shown="기본" w468 {
                  selector: w468 -> [w482 _]
                  tunnel: w472 -> [w493 _]
                  tunnel: [w491 TRUE] -> w469
                  tunnel: w471 -> [w490 _]
                  tunnel: [w479 string[] ["Zero", "0"]] -> w470
                  frame Default {
                    w485 = string[] ["", "", "", ""]
                    n133 = Index Array(array=w490, index #1=2 ("인덱스"), index #3=13 ("인덱스"), index #4=15 ("인덱스"), index #6=19 ("인덱스")) -> (element #1=w483:string, element #2=w489:string, element #3=w481:string, element #4=w480:string, element #5=w487:string, element #6=w478:string, element #7=w477:string, element #8=w476:string, element #9=w475:string, element #10=w474:string, element #11=w473:string)  [unwired: 7 in]
                    n134 = case shown="기본" w489 {
                      selector: w489 -> [w494 _]
                      tunnel: w493 -> [w500 _]
                      tunnel: w481 -> [w499 w503]
                      tunnel: [w496 w501] -> w491
                      tunnel: w482 -> [w495 w502]
                      frame Default {
                        n135 = Equal?(x=w495, y=w499) -> (x = y?=w497:bool)
                        n136 = Equal?(x=w500, y=w494) -> (x = y?=w498:bool)
                        n137 = Compound Arithmetic op=AND(w497, w498) -> (w496:bool)
                      }
                      frame "" {
                        n138 = Equal?(x=w502, y=w503) -> (x = y?=w501:bool)
                      }
                    }
                    n139 = Build Array (concatenate)(w483, w481, w487, w480, w474, w473, w481, w485, w480, w485, w478, w477, w476, w475) -> (w479:string[])
                  }
                  frame "0" {
                  }
                }
              }
              n140 = Index Array(array=w463) -> (element #1=w465:string, element #2=w464:string)  [unwired: 2 in]
              n141 = Build Array(w465, w464) -> (w462:string[])
            }
          }
          frame "Coating Thickness Specimen", "Ultrasonic Thickness Specimen" {
            n142 = Index Array(array=w529, index (col) #1=0 ("비활성화된 인덱스 (열)")) -> (element #1=w527:string[], element #2=w526:string[])  [unwired: 3 in]
            n143 = call "STD Filter.vi"("Cal STD in"=w525, "문자열(option, STD)"="Ultrasonic Thickness Specimen" ("검색 문자열")) -> ("Cal STD out"=w522:string[][], "DATA 출력"=w524:string[][])  [unwired: 5 in, 3 out]
            n144 = call "STD Filter.vi"("Cal STD in"=w522, "문자열(option, STD)"="Coating Thickness Specimen" ("검색 문자열")) -> ("Cal STD out"=w511:string[][], "DATA 출력"=w523:string[][])  [unwired: 5 in, 3 out]
            n145 = call "STD Filter.vi"("Cal STD in"=w511, "문자열(option, STD)"="Surface Plate" ("검색 문자열")) -> ("DATA 출력"=w518:string[][])  [unwired: 5 in, 4 out]
            n146 = Build Array (concatenate)(w524, w523) -> (w530:string[][])
            n147 = for {
              tunnel: w520 -> [w539] mode=indexing
              tunnel: w527 -> [w541] mode=indexing
              tunnel: w526 -> [w543] mode=indexing
              tunnel: "mm" ("환산단위") -> [w544]
              tunnel: [w537] -> w533 mode=indexing
              tunnel: w530 -> [w542]
              tunnel: [w536] -> w532 mode=indexing
              n148 = Index Array(array=w539) -> (element=w538:string)  [unwired: 1 in]
              n149 = call "Unit Conversion.vi"("환산단위"=w544, "입력단위"=w543, "입력값"=w541) -> ("환산값 (string)"=w540:string)  [unwired: 3 in, 5 out]
              n150 = for {
                tunnel: w542 -> [w548] mode=indexing
                tunnel: w538 -> [w549]
                tunnel: w540 -> [w545]
                tunnel: [w547] -> w537 if=w546
                stop <- w546 stop-if-true
                n151 = case shown="기본" w545 {
                  selector: w545 -> [w558 _]
                  tunnel: w549 -> [w567 _]
                  tunnel: [w565 TRUE] -> w546
                  tunnel: w548 -> [w564 _]
                  tunnel: [w555 string[] ["Zero", "0"]] -> w547
                  frame Default {
                    n152 = Index Array(array=w564, index #1=2 ("인덱스"), index #3=13 ("인덱스"), index #4=15 ("인덱스"), index #6=19 ("인덱스")) -> (element #1=w559:string, element #2=w563:string, element #3=w557:string, element #4=w556:string, element #5=w550:string, element #6=w554:string, element #7=w553:string, element #8=w552:string, element #9=w551:string)  [unwired: 5 in]
                    n153 = case shown="기본" w563 {
                      selector: w563 -> [w568 _]
                      tunnel: w567 -> [w574 _]
                      tunnel: w557 -> [w573 w577]
                      tunnel: [w570 w575] -> w565
                      tunnel: w558 -> [w569 w576]
                      frame Default {
                        n154 = Equal?(x=w569, y=w573) -> (x = y?=w571:bool)
                        n155 = Equal?(x=w574, y=w568) -> (x = y?=w572:bool)
                        n156 = Compound Arithmetic op=AND(w571, w572) -> (w570:bool)
                      }
                      frame "" {
                        n157 = Equal?(x=w576, y=w577) -> (x = y?=w575:bool)
                      }
                    }
                    n158 = Build Array(w559, w557, w550, w556, w550, w554, w553, w552, w551) -> (w555:string[])
                  }
                  frame "0" {
                  }
                }
              }
              n159 = Array Subset(array=w537, length=5 ("길이")) -> (w536:string[])  [unwired: 1 in]
            }
            n160 = call "Variables Data IO.vi"("Write blank data ?(F)"=TRUE ("Write blank data ?(T)"), "Select"=Cmd_Var_Data_IO."STD2", "error in"=w514, "Data In"=w518, "Func_ext"=w512) -> ("error out"=w513:errorcluster)  [unwired: 4 in, 2 out]
          }
          frame "Dial Gauge Tester" {
            n161 = call "Match_Proc_STD Unit.vi"("Cal STD 입력"=w589, "Condition Default"=w585) -> ("Cal STD 출력"=w582:string[][], "Unit"=w581:string, "Condition Default out"=w580:string[][], "STD ≥ DUT?"=w583:bool, "x < 0?"=w584:bool)  [unwired: 5 in]
            n162 = case shown="참" w583 {
              tunnel: w588 -> [_ w599]
              tunnel: [_ w601] -> w591
              tunnel: w582 -> [_ w597]
              tunnel: w581 -> [_ w596]
              tunnel: w580 -> [_ w595]
              tunnel: w584 -> [_ w594]
              frame False {
              }
              frame True {
                n163 = call "Match_Linear.vi"("기준기명"=w599, "열팽창계수(etc)"="0.0000115" ("원소"), "0보다 작음?"=w594, "환산단위(불확도)"="μm" ("환산단위"), "Cal STD in"=w597, "환산단위(교정값)"=w596, "Condition Default"=w595) -> ("Data out"=w601:string[][])  [unwired: 3 in, 1 out]
              }
            }
            n164 = Array Subset(array=w591, index (col)=0 ("인덱스"), length (col)=4 ("길이")) -> (w590:string[][])  [unwired: 2 in]
          }
          frame "Standard Scale" {
            n165 = call "STD Filter.vi"("Cal STD in"=w607, "문자열(option, STD)"=w606) -> ("DATA 출력"=w609:string[][], "문자열(option, STD)"=w608:string)  [unwired: 5 in, 3 out]
            n166 = Index Array(array=w609, index (col)=1 ("비활성화된 인덱스 (열)")) -> (element=w619:string[])  [unwired: 1 in]
            n167 = call-poly "Array Deduplication.vi"("배열 in"=w619) -> ("배열 out"=w617:string[])  [unwired: 9 in, 1 out]
            n168 = for {
              tunnel: w617 -> [w626] mode=indexing
              tunnel: w609 -> [w627]
              tunnel: [w621] -> w618 mode=indexing
              n169 = call-poly "Data Classification.vi"("인덱스"=1, "DATA 입력"=w627, "검색 문자열"=w626) -> ("DATA 출력"=w625:string[][])  [unwired: 4 in, 4 out]
              n170 = Index Array(array=w625, index (col)=13 ("비활성화된 인덱스 (열)")) -> (element=w623:string[])  [unwired: 1 in]
              n171 = Fract/Exp String To Number(string=w623) -> (number=w622:dbl[])  [unwired: 3 in, 1 out]
              n172 = Array Max & Min(array=w622) -> (max value=w621:dbl)  [unwired: 3 out]
            }
            n173 = Array Max & Min(array=w618) -> (max index (indices)=w616:i32)  [unwired: 3 out]
            n174 = Index Array(array=w617, index=w616) -> (element=w615:string)
            n175 = call-poly "Data Classification.vi"("인덱스"=1, "DATA 입력"=w609, "검색 문자열"=w615) -> ("DATA 출력"=w611:string[][])  [unwired: 4 in, 4 out]
            n176 = call "Match_Linear.vi"("절대값?"=TRUE, "기준기명"=w608, "열팽창계수(etc)"="0.000008" ("열팽창계수"), "환산단위(불확도)"="μm" ("환산단위2"), "Cal STD in"=w611, "환산단위(교정값)"="mm" ("환산단위1"), "Condition Default"=w604) -> ("Data out"=w605:string[][])  [unwired: 3 in, 1 out]
          }
          frame "Gauge Block" {
            n177 = call "Match_Gauge Block.vi"("Calibration Default"=w631, "세부분류코드"=w632, "Cal STD"=w630, "에러 입력"=w637, "Func_ext in"=w629) -> ("에러 출력"=w633:errorcluster, "Data Out 2"=w634:string[], "Data Out"=w635:string[][], "CalSTD"=w636:string[][])  [unwired: 3 in]
          }
          frame "Laser Extensometer" {
            n178 = call "Match_Proc_STD Unit.vi"("Cal STD 입력"=w645, "Condition Default"=w642) -> ("Cal STD 출력"=w640:string[][], "Unit"=w639:string, "Condition Default out"=w638:string[][], "STD ≥ DUT?"=w641:bool)  [unwired: 5 in, 1 out]
            n179 = case shown="참" w641 {
              tunnel: [_ w658] -> w649
              tunnel: w646 -> [_ w656]
              tunnel: w640 -> [_ w654]
              tunnel: w639 -> [_ w653]
              tunnel: w638 -> [_ w651]
              frame False {
              }
              frame True {
                n180 = call "Match_Linear.vi"("절대값?"=TRUE, "기준기명"=w656, "열팽창계수(etc)"="0" ("원소"), "환산단위(불확도)"="μm" ("환산단위"), "Cal STD in"=w654, "환산단위(교정값)"=w653, "Condition Default"=w651) -> ("Data out"=w658:string[][])  [unwired: 3 in, 1 out]
              }
            }
            n181 = Array Subset(array=w649, index (col)=0 ("인덱스"), length (col)=4 ("길이")) -> (w648:string[][])  [unwired: 2 in]
          }
          frame "Laser Interferometer" {
            n182 = case shown="\"10227-0\", \"10413-0\"" w663 {
              tunnel: [w683 w709] -> w670
              tunnel: w668 -> [w688 w708]
              tunnel: w665 -> [w673 w707]
              tunnel: w664 -> [w689 w704]
              tunnel: [string[] ["기준기명", "명목값", "단위"] string[] ["기준기명", "명목값", "단위", "교정값"]] -> w662
              tunnel: [w676 w705] -> w661
              tunnel: w660 -> [w677 w705]
              tunnel: w659 -> [w675 _]
              frame "10227-0", "10413-0" {
                n183 = call "STD Filter.vi"("Cal STD in"=w673, "문자열(option, STD)"="Tape Measure Calibration System" ("검색 문자열")) -> ("DATA 출력"=w672:string[][])  [unwired: 5 in, 4 out]
                n184 = Index Array(array=w673, index (row) #1=0 ("인덱스 (행)"), index (col) #1=19 ("비활성화된 인덱스 (열)")) -> (element #1=w684:string, element #2=w682:string, element #3=w681:string, element #4=w680:string, element #5=w679:string)  [unwired: 8 in]
                n185 = call "Variables Data IO.vi"("Write blank data ?(F)"=TRUE ("Write blank data ?(T)"), "Select"=Cmd_Var_Data_IO."STD2", "error in"=w677, "Data In"=w672, "Func_ext"=w675) -> ("error out"=w676:errorcluster)  [unwired: 4 in, 2 out]
                n186 = for {
                  tunnel: w689 -> [w699] mode=indexing
                  tunnel: w688 -> [w698]
                  tunnel: w684 -> [w695]
                  tunnel: [w694] -> w683 mode=indexing
                  tunnel: w682 -> [w693]
                  tunnel: w681 -> [w692]
                  tunnel: w680 -> [w691]
                  tunnel: w679 -> [w690]
                  n187 = Index Array(array=w699) -> (element #1=w697:string, element #2=w696:string)  [unwired: 2 in]
                  n188 = Build Array(w698, w697, w696, w695, w693, w692, w691, w690) -> (w694:string[])
                }
              }
              frame Default {
                n189 = call "Match_Proc_STD Unit.vi"("Cal STD 입력"=w707, "Condition Default"=w704) -> ("Cal STD 출력"=w702:string[][], "Unit"=w701:string, "Condition Default out"=w700:string[][], "STD ≥ DUT?"=w703:bool)  [unwired: 5 in, 1 out]
                n190 = case shown="참" w703 {
                  tunnel: [_ w710] -> w709
                  tunnel: w708 -> [_ w711]
                  tunnel: w702 -> [_ w714]
                  tunnel: w701 -> [_ w715]
                  tunnel: w700 -> [_ w716]
                  frame False {
                  }
                  frame True {
                    n191 = call "Match_Linear.vi"("기준기명"=w711, "열팽창계수(etc)"="0.0000115" ("원소"), "환산단위(불확도)"="μm" ("환산단위"), "Cal STD in"=w714, "환산단위(교정값)"=w715, "Condition Default"=w716) -> ("Data out"=w710:string[][])  [unwired: 4 in, 1 out]
                  }
                }
              }
            }
            n192 = Array Subset(array=w670, index (col)=0 ("인덱스"), length (col)=3 ("길이")) -> (w669:string[][])  [unwired: 2 in]
          }
          frame Default {
          }
        }
      }
      n193 = Index Array(array=w413) -> (element=w415:string[])  [unwired: 2 in]
      n194 = call "Match_Cal STD.vi"("Condition Default"=w416, "Data 2 in"=w413, "Data in"=w417, "Cal STD"=w420) -> ("Data Out"=w418:string[][], "Cal STD"=w419:string[][])  [unwired: 5 in, 1 out]
    }
    frame "Length_10" {
      w719 = 0 ("인덱스 (행)")
      w760 = 2 ("인덱스")
      w736 = i32[] [1, 2, 14, 17, 16, 19, 21, 22]
      n195 = Array Subset(array=w761, index (col)=w760, length (col)=w760) -> (w734:string[][])  [unwired: 2 in]
      n196 = Index Array(array=w732, index (row) #1=w719, index (col) #1=w719, index (row) #2=1 ("비활성화된 인덱스 (행)"), index (col) #2=w719) -> (element #1=w718:string, element #2=w726:string, element #3=w731:string, element #4=w730:string)  [unwired: 4 in]
      n197 = call "STD Filter.vi"("Cal STD in"=w733, "STD select"=Cmd_STD_select."DMM", "Condition"=w734) -> ("DATA 출력"=w747:string[][])  [unwired: 4 in, 4 out]
      n198 = for {
        tunnel: w747 -> [w769] mode=indexing
        tunnel: w736 -> [w770]
        tunnel: [w768] -> w745 mode=indexing
        n199 = for {
          tunnel: w770 -> [w771] mode=indexing
          tunnel: w769 -> [w772]
          tunnel: [w773] -> w768 mode=indexing
          n200 = Index Array(array=w772, index=w771) -> (element=w773:string)
        }
      }
      n201 = call "Unit Conversion.vi"("환산단위"="kHz", "입력단위"=w730, "입력값"=w731) -> ("환산값 (string)"=w728:string)  [unwired: 3 in, 5 out]
      n202 = Equal?(x=w726, y="DC") -> (x = y?=w725:bool)
      n203 = call "Variables Data IO.vi"("Write blank data ?(F)"=TRUE ("Write blank data ?(T)"), "Select"=Cmd_Var_Data_IO."STD2", "error in"=w757, "Data In"=w745, "Func_ext"=w759) -> ("error out"=w739:errorcluster, "Func_ext Out"=w740:string)  [unwired: 4 in, 1 out]
      n204 = Select(t=Cmd_STD_select."Power Supply" ("STD select"), s=w725, f=Cmd_STD_select."Calibrator" ("STD select")) -> (s? t:f=w721:T4)
      n205 = call "STD Filter.vi"("Cal STD in"=w733, "STD select"=w721, "문자열(option, STD)"=w728, "Condition"=w734, "값(option)"=w718) -> ("DATA 출력"=w724:string[][])  [unwired: 2 in, 4 out]
      n206 = for {
        tunnel: w724 -> [w763] mode=indexing
        tunnel: w736 -> [w764]
        tunnel: [w762] -> w741 mode=indexing
        n207 = for {
          tunnel: w764 -> [w765] mode=indexing
          tunnel: w763 -> [w766]
          tunnel: [w767] -> w762 mode=indexing
          n208 = Index Array(array=w766, index=w765) -> (element=w767:string)
        }
      }
      n209 = call "Variables Data IO.vi"("Write blank data ?(F)"=TRUE ("Write blank data ?(T)"), "Select"=Cmd_Var_Data_IO."STD3", "error in"=w739, "Data In"=w741, "Func_ext"=w740) -> ("error out"=w737:errorcluster, "Func_ext Out"=w738:string)  [unwired: 4 in, 1 out]
      n210 = for {
        tunnel: [w785] -> w753 mode=indexing
        tunnel: [w784] -> w755 mode=indexing
        tunnel: [w783] -> w751 mode=indexing
        tunnel: w758 -> [w782]
        tunnel: w738 -> [w778]
        tunnel: w733 -> [w777]
        shift-right: [w780] -> w756
        shift-left: w737 -> [w779]
        tunnel: w748 -> [w776] mode=indexing
        tunnel: w749 -> [w781]
        n211 = call "STD Filter.vi"("Cal STD in"=w777, "문자열(option, STD)"=w776) -> ("DATA 출력"=w775:string[][], "문자열(option, STD)"=w774:string)  [unwired: 5 in, 3 out]
        n212 = case shown="\"Dial Gauge Tester\"" w774 {
          selector: w774 -> [_ _ w812]
          tunnel: [_ w796 w806] -> w785
          tunnel: [w787 w795 w805] -> w784
          tunnel: [_ w794 string[] ["기준기명", "명목값", "단위", "교정값", "단위"] ("Data Out 2")] -> w783
          tunnel: w782 -> [_ w793 _]
          tunnel: w781 -> [_ w788 w813]
          tunnel: [w786 w792 w814] -> w780
          tunnel: w779 -> [w786 w791 w814]
          tunnel: w778 -> [_ w790 _]
          tunnel: w775 -> [w787 w789 w811]
          frame Default {
          }
          frame "Gauge Block" {
            n213 = call "Match_Gauge Block.vi"("Calibration Default"=w788, "세부분류코드"=w793, "Cal STD"=w789, "에러 입력"=w791, "Func_ext in"=w790) -> ("에러 출력"=w792:errorcluster, "Data Out 2"=w794:string[], "Data Out"=w796:string[][], "CalSTD"=w795:string[][])  [unwired: 3 in]
          }
          frame "Dial Gauge Tester" {
            n214 = call "Match_Proc_STD Unit.vi"("Cal STD 입력"=w811, "Condition Default"=w813) -> ("Cal STD 출력"=w799:string[][], "Unit"=w800:string, "Condition Default out"=w797:string[][], "STD ≥ DUT?"=w801:bool, "x < 0?"=w798:bool)  [unwired: 5 in]
            n215 = case shown="참" w801 {
              tunnel: w812 -> [_ w820]
              tunnel: [_ w822] -> w805
              tunnel: w799 -> [_ w818]
              tunnel: w800 -> [_ w817]
              tunnel: w797 -> [_ w816]
              tunnel: w798 -> [_ w815]
              frame False {
              }
              frame True {
                n216 = call "Match_Linear.vi"("기준기명"=w820, "열팽창계수(etc)"="0.0000115" ("원소"), "0보다 작음?"=w815, "환산단위(불확도)"="μm" ("환산단위"), "Cal STD in"=w818, "환산단위(교정값)"=w817, "Condition Default"=w816) -> ("Data out"=w822:string[][])  [unwired: 3 in, 1 out]
              }
            }
            n217 = Index Array(array=w805, index (col) #1=12 ("비활성화된 인덱스 (열)")) -> (element #1=w803:string[])  [unwired: 3 in, 1 out]
            n218 = Array Subset(array=w805, index (col)=0 ("인덱스"), length (col)=5 ("길이")) -> (w807:string[][])  [unwired: 2 in]
            n219 = Replace Array Subset(array=w807, new element=w803, index (col)=2 ("비활성화된 인덱스 (열)")) -> (w806:string[][])  [unwired: 1 in]
          }
        }
      }
      n220 = call "Match_Cal STD.vi"("Condition Default"=w749, "Data 2 in"=w751, "Data in"=w753, "Cal STD"=w755) -> ("Data 2 Out"=w750:string[], "Data Out"=w752:string[][], "Cal STD"=w754:string[][])  [unwired: 5 in]
    }
    frame "Length_11" {
      n221 = Index Array(array=w823, index=0 ("인덱스 (행)")) -> (element=w831:string)
      n222 = Index Array(array=w824, index (col) #1=0 ("비활성화된 인덱스 (열)")) -> (element #1=w835:string[], element #2=w834:string[])  [unwired: 3 in]
      n223 = case shown="\"Bench Micrometer\"" w831 {
        tunnel: ["Analog(1/2)" "Digital" "Digital"] -> w830
        tunnel: ["μm" ("환산단위") "mm" ("환산단위") "μm" ("환산단위")] -> w829
        tunnel: w828 -> [_ w841 _]
        tunnel: w827 -> [_ w848 _]
        tunnel: w826 -> [w838 w847 w852]
        tunnel: [w838 w846 w852] -> w825
        frame "Bench Micrometer" {
        }
        frame "Measuring Projector" {
          n224 = call "STD Filter.vi"("Cal STD in"=w841, "STD select"=Cmd_STD_select."Measuring Projector", "문자열(option, STD)"="Magnification" ("검색 문자열")) -> ("DATA 출력"=w842:string[][])  [unwired: 4 in, 4 out]
          n225 = call "Variables Data IO.vi"("Write blank data ?(F)"=TRUE ("Write blank data ?(T)"), "Select"=Cmd_Var_Data_IO."STD2", "error in"=w847, "Data In"=w842, "Func_ext"=w848) -> ("error out"=w846:errorcluster)  [unwired: 4 in, 2 out]
        }
        frame Default {
        }
      }
      n226 = for {
        tunnel: w828 -> [w894]
        tunnel: [w891] -> w837 mode=indexing
        tunnel: [w869] -> w836 mode=indexing
        tunnel: w835 -> [w865] mode=indexing
        tunnel: w834 -> [w864] mode=indexing
        tunnel: w830 -> [w863]
        tunnel: w829 -> [w856]
        w862 = 0 ("인덱스 (열)")
        n227 = Index Array(array=w894, index (row) #1=w862, index (col) #1=16 ("비활성화된 인덱스 (열)"), index (row) #2=w862, index (col) #2=1 ("비활성화된 인덱스 (열)"), index (col) #4=13 ("인덱스 (행)"), index (col) #5=17 ("인덱스 (행)"), index (row) #6=w862, index (col) #6=18 ("인덱스 (행)")) -> (element #1=w860:string, element #2=w858:string, element #3=w857:string, element #4=w880:string[], element #5=w878:string[], element #6=w875:string, element #7=w889:string, element #8=w882:string, element #9=w883:string, element #10=w877:string, element #11=w872:string, element #12=w868:string, element #13=w870:string)  [unwired: 18 in]
        n228 = call "Unit Conversion.vi"("환산단위"=w860, "입력단위"=w864, "입력값"=w865) -> ("환산값 (DBL)"=w887:dbl)  [unwired: 3 in, 5 out]
        n229 = Fract/Exp String To Number(string=w880) -> (number=w890:dbl[])  [unwired: 3 in, 1 out]
        n230 = Fract/Exp String To Number(string=w878) -> (number=w893:dbl[])  [unwired: 3 in, 1 out]
        n231 = Threshold 1D Array(2:w887, 3:w890) -> (0:w888:dbl)  [unwired: 1 in]
        n232 = call "Unit Conversion.vi"("환산단위"="μm", "입력단위"=w883, "입력값"=w889) -> ("환산단위"=w884:string, "환산값 (string)"=w885:string)  [unwired: 3 in, 4 out]
        n233 = call "Unit Conversion.vi"("환산단위"=w864, "입력단위"=w856, "입력값"=w868) -> ("환산단위"=w866:string, "환산값 (string)"=w867:string)  [unwired: 3 in, 4 out]
        n234 = Interpolate 1D Array(1:w888, 2:w893) -> (0:w892:dbl)
        n235 = Format Into String(format string="%#.2g" ("포맷 문자열"), w892) -> (resulting string=w876:string)  [unwired: 2 in, 1 out]
        n236 = Build Array(w863, w867, w866) -> (w869:string[])
        n237 = call "Unit Conversion.vi"("환산단위"=w864, "입력단위"=w875, "입력값"=w876) -> ("환산단위"=w873:string, "환산값 (string)"=w874:string)  [unwired: 3 in, 4 out]
        n238 = Build Array(w858, w857, w865, w864, w874, w873, w885, w882, w884, w877, w872, w868, w870) -> (w891:string[])
      }
    }
    frame "Length_12" {
      n239 = call "Match_Gauge Block.vi"("Data in"=w896, "Calibration Default"=w895, "세부분류코드"=w901, "Cal STD"=w899, "에러 입력"=w898, "Func_ext in"=w900) -> ("에러 출력"=w897:errorcluster, "Data Out 2"=w902:string[], "Data Out"=w903:string[][], "CalSTD"=w904:string[][])  [unwired: 2 in]
    }
    frame "Length_13" {
      w928 = FALSE ("교정(T) 보정(F)")
      w910 = "0.0000085" ("열팽창계수")
      w911 = "μm" ("환산단위2")
      w912 = "mm" ("환산단위1")
      n240 = call "STD Filter.vi"("Cal STD in"=w917, "STD select"=Cmd_STD_select."Ring Gauge", "문자열(option, STD)"=w913) -> ("DATA 출력"=w918:string[][])  [unwired: 4 in, 4 out]
      n241 = Search/Split String(string=w913, search string/char (-)=" " ("검색 문자열/문자 (-)")) -> (substring before match=w927:string, match + rest of string=w934:string)  [unwired: 1 in, 1 out]
      n242 = Index Array(array=w918) -> (element=w929:string[])  [unwired: 2 in]
      n243 = call "Variables Data IO.vi"("Write blank data ?(F)"=TRUE ("Write blank data ?(T)"), "Select"=Cmd_Var_Data_IO."STD2", "error in"=w931, "Data In"=w918, "Func_ext"=w930) -> ("error out"=w922:errorcluster, "Func_ext Out"=w920:string)  [unwired: 4 in, 1 out]
      n244 = call <vilib>:"Trim Whitespace.vi"("string"=w934) -> ("trimmed string"=w926:string)  [unwired: 1 in]
      n245 = call "STD Filter.vi"("Cal STD in"=w917, "문자열(option, STD)"="Standard Measuring Machine" ("검색 문자열")) -> ("DATA 출력"=w909:string[][], "문자열(option, STD)"=w906:string)  [unwired: 5 in, 3 out]
      n246 = Build Array(w927, w926) -> (w925:string[])
      n247 = Index Array(array=w909, index (row)=0 ("비활성화된 인덱스 (행)"), index (col)=24 ("비활성화된 인덱스 (열)")) -> (element=w937:string)
      n248 = Build Array(w925) -> (w915:string[][])
      n249 = call "Match_Linear.vi"("기준기명"=w906, "교정(T) 보정(F)"=w928, "열팽창계수(etc)"=w910, "환산단위(불확도)"=w911, "Cal STD in"=w909, "환산단위(교정값)"=w912, "Condition Default"=w915) -> ("Cal STD out"=w905:string[][], "Data out"=w916:string[][])  [unwired: 3 in]
      n250 = call "Match_Linear.vi"("기준기명"=w906, "교정(T) 보정(F)"=w928, "열팽창계수(etc)"=w910, "환산단위(불확도)"=w911, "Cal STD in"=w905, "환산단위(교정값)"=w912, "Condition Default"=w914) -> ("Data out"=w908:string[][])  [unwired: 3 in, 1 out]
      n251 = for {
        tunnel: w937 -> [w944]
        tunnel: [w945] -> w936 mode=indexing
        tunnel: w908 -> [_] mode=indexing
        n252 = call "Unit Conversion.vi"("환산단위"="mm", "입력단위"="μm" ("원소"), "입력값"=w944) -> ("환산단위"=w940:string, "환산값 (string)"=w941:string)  [unwired: 3 in, 4 out]
        n253 = Build Array("Digital" ("원소"), w941, w940) -> (w945:string[])
      }
      n254 = call "Variables Data IO.vi"("Write blank data ?(F)"=TRUE ("Write blank data ?(T)"), "Select"=Cmd_Var_Data_IO."STD3", "error in"=w922, "Data In"=w916, "Func_ext"=w920) -> ("error out"=w921:errorcluster)  [unwired: 4 in, 2 out]
    }
    frame "Length_14" {
      w954 = 0 ("비활성화된 인덱스 (열)")
      w966 = 13 ("비활성화된 인덱스 (열)")
      # "dw=p/2*1/cos(a/2)"
      n255 = call "STD Filter.vi"("Cal STD in"=w982, "문자열(option, STD)"="Thread Measuring Wire Gauge") -> ("제외 DATA 출력"=w973:string[][], "Cal STD out"=w971:string[][], "DATA 출력"=w968:string[][])  [unwired: 5 in, 2 out]
      n256 = call "STD Filter.vi"("Cal STD in"=w973, "문자열(option, STD)"="Gauge Block") -> ("DATA 출력"=w972:string[][])  [unwired: 5 in, 4 out]
      n257 = Index Array(array=w983, index (col)=1 ("비활성화된 인덱스 (열)")) -> (element=w970:string[])  [unwired: 1 in]
      n258 = call "Variables Data IO.vi"("Write blank data ?(F)"=TRUE, "Select"=Cmd_Var_Data_IO."STD3", "error in"=w980, "Data In"=w972, "Func_ext"=w978) -> ("error out"=w962:errorcluster, "Func_ext Out"=w975:string)  [unwired: 4 in, 1 out]
      n259 = for {
        tunnel: w970 -> [w1018] mode=indexing
        tunnel: w957 -> [w1009] mode=indexing
        tunnel: w971 -> [w1019]
        tunnel: [w1008] -> w984 mode=indexing
        n260 = case shown="\"바깥지름\", \"유효지름\", 기본" w1018 {
          tunnel: w1019 -> [w1028 w1037 w1047]
          tunnel: w1009 -> [w1026 w1036 w1046]
          tunnel: [w1025 w1030 w1040] -> w1017
          tunnel: ["0.000008" ("환산단위2") "0.000008" ("환산단위2") "0.000008" ("환산단위2")] -> w1015
          tunnel: [w1020 w1029 w1038] -> w1014
          tunnel: [w1023 w1033 w1043] -> w1013
          tunnel: ["mm" ("환산단위1") "mm" ("환산단위1") "˚" ("환산단위1")] -> w1012
          tunnel: [w1021 w1034 w1044] -> w1011
          tunnel: [w1020 w1029 w1038] -> w1007
          frame "바깥지름", "유효지름", Default {
            w1020 = "μm" ("환산단위2")
            n261 = Build Array(w1026) -> (w1021:string[][])
            n262 = call "STD Filter.vi"("Cal STD in"=w1028, "문자열(option, STD)"="Standard Measuring Machine" ("검색 문자열")) -> ("DATA 출력"=w1023:string[][], "문자열(option, STD)"=w1025:string)  [unwired: 5 in, 3 out]
          }
          frame "피치" {
            w1029 = "μm" ("환산단위2")
            n263 = Build Array(w1036) -> (w1034:string[][])
            n264 = call "STD Filter.vi"("Cal STD in"=w1037, "STD select"=Cmd_STD_select."Measuring Projector") -> ("DATA 출력"=w1033:string[][], "문자열(option, STD)"=w1030:string)  [unwired: 5 in, 3 out]
          }
          frame "산의반각" {
            w1038 = "´" ("환산단위2")
            n265 = Build Array(w1046) -> (w1044:string[][])
            n266 = call "STD Filter.vi"("Cal STD in"=w1047, "STD select"=Cmd_STD_select."Measuring Projector", "문자열(option, STD)"="Angle") -> ("DATA 출력"=w1043:string[][], "문자열(option, STD)"=w1040:string)  [unwired: 4 in, 3 out]
          }
        }
        n267 = call "Match_Linear.vi"("환산단위(보정값)"=w1007, "기준기명"=w1017, "교정(T) 보정(F)"=FALSE, "열팽창계수(etc)"=w1015, "환산단위(불확도)"=w1014, "Cal STD in"=w1013, "환산단위(교정값)"=w1012, "Condition Default"=w1011) -> ("Data out"=w1010:string[][])  [unwired: 2 in, 1 out]
        n268 = Index Array(array=w1010) -> (element=w1008:string[])  [unwired: 2 in]
      }
      n269 = Index Array(array=w957, index (row) #1=3 ("인덱스 (행)"), index (col) #1=w954, index (row) #2=10 ("비활성화된 인덱스 (열)"), index (col) #2=w954) -> (element #1=w955:string, element #2=w952:string)
      n270 = Fract/Exp String To Number(string=w955) -> (number=w958:dbl)  [unwired: 3 in, 1 out]
      n271 = Fract/Exp String To Number(string=w952) -> (number=w951:dbl)  [unwired: 3 in, 1 out]
      n272 = Multiply(x=w951, y=2.0) -> (x*y=w950:dbl)
      n273 = call "Thread_dw.vi"("α"=w950, "P"=w958) -> ("결과"=w948:dbl)  [unwired: 1 in, 1 out]
      n274 = case shown="\"가까운 값\"" w947 {
        tunnel: w968 -> [w986 w999]
        tunnel: [w988 w998] -> w963
        tunnel: w948 -> [w987 w997]
        frame "가까운 값" {
          n275 = for {
            tunnel: w986 -> [w996] mode=indexing
            tunnel: w987 -> [w994]
            tunnel: [w991] -> w989 mode=indexing
            n276 = Index Array(array=w996, index=13 ("인덱스")) -> (element=w995:string)
            n277 = Fract/Exp String To Number(string=w995) -> (number=w993:dbl)  [unwired: 3 in, 1 out]
            n278 = Subtract(x=w994, y=w993) -> (x-y=w992:dbl)
            n279 = Absolute Value(x=w992) -> (abs(x)=w991:dbl)
          }
          n280 = Array Max & Min(array=w989) -> (min index (indices)=w988:i32)  [unwired: 3 out]
        }
        frame "큰 값", Default {
          n281 = for {
            tunnel: w999 -> [w1006] mode=indexing
            tunnel: w997 -> [w1002]
            tunnel: [w1000] -> w998
            i -> [w1000]
            stop <- w1001 stop-if-true
            n282 = Index Array(array=w1006, index=13 ("인덱스")) -> (element=w1005:string)
            n283 = Fract/Exp String To Number(string=w1005) -> (number=w1003:dbl)  [unwired: 3 in, 1 out]
            n284 = Greater Or Equal?(x=w1003, y=w1002) -> (x >= y?=w1001:bool)
          }
        }
      }
      n285 = Index Array(array=w968, index (row) #1=w963, index (col) #1=w966, index (col) #2=w966) -> (element #1=w969:string, element #2=w965:string[])  [unwired: 1 in]
      n286 = call-poly "Array Deduplication.vi"("error in (no error)"=w962, "배열 in"=w965) -> ("error out"=w960:errorcluster, "배열 out"=w964:string[])  [unwired: 8 in]
      n287 = call-poly "Data Classification.vi"("인덱스"=w966, "DATA 입력"=w968, "검색 문자열"=w969) -> ("DATA 출력"=w967:string[][])  [unwired: 4 in, 4 out]
      n288 = call "Variables Data IO.vi"("Write blank data ?(F)"=TRUE, "Select"=Cmd_Var_Data_IO."STD2", "error in"=w960, "Data In"=w967, "Func_ext"=w975) -> ("error out"=w961:errorcluster)  [unwired: 4 in, 2 out]
    }
    frame "Length_15" {
      w1052 = 0 ("인덱스 (행)")
      n289 = Index Array(array=w1053, index (row)=w1052, index (col)=w1052) -> (element=w1051:string)
      n290 = call-poly "Data Classification.vi"("인덱스"=24, "DATA 입력"=w1050, "검색 문자열"=w1051) -> ("DATA 출력"=w1049:string[][])  [unwired: 4 in, 4 out]
    }
    frame "Length_16" {
      w1065 = 0 ("인덱스 (행)")
      n291 = Index Array(array=w1067, index (row) #1=w1065, index (col) #1=2 ("비활성화된 인덱스 (열)"), index (row) #2=w1065, index (col) #2=24 ("비활성화된 인덱스 (열)")) -> (element #1=w1062:string, element #2=w1063:string, element #3=w1056:string)  [unwired: 2 in]
      n292 = case shown="\"Standard Measuring Machine\"" w1062 {
        selector: w1062 -> [w1074 w1077 w1080]
        tunnel: ["0.0000115" ("열팽창계수") "0.0000115" ("열팽창계수") "0.0000085" ("열팽창계수")] -> w1061
        tunnel: [w1074 w1077 w1080] -> w1060
        tunnel: ["Digital" ("원소") "Analog" ("원소") "Digital" ("원소")] -> w1059
        frame Default {
        }
        frame "Bench Micrometer" {
        }
        frame "Standard Measuring Machine" {
        }
      }
      n293 = call "Match_Linear.vi"("기준기명"=w1060, "교정(T) 보정(F)"=FALSE, "열팽창계수(etc)"=w1061, "환산단위(불확도)"="μm" ("환산단위2"), "Cal STD in"=w1067, "환산단위(교정값)"="mm" ("환산단위1"), "Condition Default"=w1068) -> ("Data out"=w1058:string[][])  [unwired: 3 in, 1 out]
      n294 = for {
        tunnel: w1063 -> [w1083]
        tunnel: [w1091] -> w1072 mode=indexing
        tunnel: w1059 -> [w1086]
        tunnel: w1058 -> [w1085] mode=indexing
        tunnel: [w1084] -> w1057 mode=indexing
        tunnel: w1056 -> [w1082]
        n295 = call "Unit Conversion.vi"("환산단위"="mm", "입력단위"="μm" ("원소"), "입력값"=w1083) -> ("환산단위"=w1087:string, "환산값 (string)"=w1088:string)  [unwired: 3 in, 4 out]
        n296 = Insert Into Array(array=w1085, new element #1=w1083, new element #2=w1082) -> (w1084:string[])  [unwired: 1 in]
        n297 = Build Array(w1086, w1088, w1087) -> (w1091:string[])
      }
    }
    frame "Length_2" {
      n298 = call "Match_Gauge Block.vi"("Calibration Default"=w1097, "세부분류코드"=w1095, "Cal STD"=w1096, "에러 입력"=w1094, "Func_ext in"=w1092) -> ("에러 출력"=w1093:errorcluster, "Data Out"=w1099:string[][], "CalSTD"=w1098:string[][])  [unwired: 3 in, 1 out]
    }
    frame "Length_3" {
      n299 = case shown="기본" w1101 {
        tunnel: w1105 -> [w1110 w1176]
        tunnel: [w1109 w1175] -> w1104
        tunnel: [w1108 w1174] -> w1103
        tunnel: w1102 -> [w1107 w1171]
        tunnel: w1100 -> [_ w1173]
        frame Default {
          n300 = for {
            tunnel: w1110 -> [w1120] mode=indexing
            tunnel: w1107 -> [w1121]
            tunnel: [w1119] -> w1109 mode=indexing
            tunnel: [w1111] -> w1108 mode=indexing
            n301 = Index Array(array=w1120) -> (element #1=w1118:string, element #2=w1115:string)  [unwired: 2 in]
            n302 = call "Unit Conversion.vi"("환산단위"="μm", "입력단위"=w1115, "입력값"=w1118) -> ("환산단위"=w1116:string, "환산값 (string)"=w1114:string)  [unwired: 3 in, 4 out]
            n303 = case shown="기본" w1114 {
              selector: w1114 -> [w1122 w1126]
              tunnel: w1121 -> [_ w1129]
              tunnel: [string[] ["0", "", "", "", "", "", "", "", "", "", "", "", "", "0", "0", "0", "", "0", "", "0"] ("t") w1124] -> w1119
              tunnel: w1116 -> [_ w1128]
              tunnel: w1115 -> [_ w1127]
              tunnel: [w1122 w1125] -> w1112
              frame "0" {
              }
              frame Default {
                n304 = for {
                  tunnel: w1129 -> [w1162] mode=indexing
                  tunnel: w1126 -> [w1160]
                  tunnel: w1128 -> [w1165]
                  tunnel: [w1134] -> w1124
                  tunnel: w1127 -> [w1143]
                  tunnel: [w1130] -> w1125
                  stop <- w1133 stop-if-true
                  n305 = Index Array(array=w1162, index #1=13 ("인덱스"), index #5=17 ("인덱스"), index #7=25 ("인덱스")) -> (element #1=w1159:string, element #2=w1155:string, element #3=w1153:string, element #4=w1144:string, element #5=w1150:string, element #6=w1149:string, element #7=w1145:string)  [unwired: 4 in]
                  n306 = Equal?(x=w1160, y=w1159) -> (x = y?=w1164:bool)
                  n307 = Equal?(x=w1165, y=w1144) -> (x = y?=w1163:bool)
                  n308 = call "Unit Conversion.vi"("환산단위"=w1143, "입력단위"=w1144, "입력값"=w1159) -> ("환산값 (string)"=w1156:string)  [unwired: 3 in, 5 out]
                  n309 = call "Unit Conversion.vi"("환산단위"=w1143, "입력단위"=w1144, "입력값"=w1155) -> ("환산값 (string)"=w1154:string)  [unwired: 3 in, 5 out]
                  n310 = call "Unit Conversion.vi"("환산단위"=w1143, "입력단위"=w1144, "입력값"=w1153) -> ("환산단위"=w1152:string, "환산값 (DBL)"=w1137:dbl, "환산값 (string)"=w1132:string)  [unwired: 3 in, 3 out]
                  n311 = call "Unit Conversion.vi"("환산단위"=w1143, "입력단위"=w1149, "입력값"=w1150) -> ("환산단위"=w1147:string, "환산값 (string)"=w1148:string)  [unwired: 3 in, 4 out]
                  n312 = call "Unit Conversion.vi"("환산단위"=w1143, "입력단위"=w1144, "입력값"=w1145) -> ("환산값 (DBL)"=w1136:dbl, "환산값 (string)"=w1141:string)  [unwired: 3 in, 4 out]
                  n313 = And(x=w1164, y=w1163) -> (x .and. y?=w1133:bool)
                  n314 = Select(t=w1162, s=w1133, f=string[] [""]) -> (s? t:f=w1158:string[])
                  n315 = Subtract(x=w1137, y=w1136) -> (x-y=w1138:dbl)
                  n316 = Select(t=w1132, s=w1133, f="") -> (s? t:f=w1130:string)
                  n317 = Absolute Value(x=w1138) -> (abs(x)=w1139:dbl)
                  n318 = Format Into String(format string="%#f" ("포맷 문자열"), w1139) -> (resulting string=w1135:string)  [unwired: 2 in, 1 out]
                  n319 = Replace Array Subset(array=w1158, new element #1=w1156, index #1=13 ("인덱스"), new element #2=w1154, new element #3=w1132, new element #4=w1152, new element #5=w1148, new element #6=w1147, new element #7=w1141, index #7=25 ("인덱스"), new element #8=w1135) -> (w1134:string[])  [unwired: 6 in]
                }
              }
            }
            n320 = Insert Into Array(array=w1120, index=1 ("인덱스"), new element=w1112) -> (w1111:string[])
          }
        }
        frame "10517-0" {
          w1172 = 0 ("인덱스 (행)")
          n321 = Index Array(array=w1173, index (row)=w1172, index (col)=w1172) -> (element=w1170:string)
          n322 = Search and Replace String(input string=w1170, search string="Pt" ("검색 문자열"), replace string="Step Height" ("검색 문자열")) -> (result string=w1169:string)  [unwired: 5 in, 3 out]
          n323 = for {
            tunnel: w1176 -> [w1187] mode=indexing
            tunnel: w1171 -> [w1188]
            tunnel: [w1186] -> w1175 mode=indexing
            tunnel: [w1179] -> w1174 mode=indexing
            tunnel: w1169 -> [w1178]
            n324 = Index Array(array=w1187) -> (element #1=w1185:string, element #2=w1182:string)  [unwired: 2 in]
            n325 = call "Unit Conversion.vi"("환산단위"="μm", "입력단위"=w1182, "입력값"=w1185) -> ("환산단위"=w1183:string, "환산값 (string)"=w1181:string)  [unwired: 3 in, 4 out]
            n326 = case shown="기본" w1181 {
              selector: w1181 -> [w1189 w1194]
              tunnel: w1188 -> [_ w1197]
              tunnel: [string[] ["0", "", "", "", "", "", "", "", "", "", "", "", "", "0", "0", "0", "", "0", "", "0"] ("t") w1192] -> w1186
              tunnel: w1183 -> [_ w1196]
              tunnel: w1182 -> [_ w1195]
              tunnel: [w1189 w1193] -> w1177
              tunnel: w1178 -> [_ w1191]
              frame "0" {
              }
              frame Default {
                n327 = for {
                  tunnel: w1197 -> [w1234] mode=indexing
                  tunnel: w1194 -> [w1232]
                  tunnel: w1196 -> [w1237]
                  tunnel: [w1229] -> w1192
                  tunnel: w1195 -> [w1214]
                  tunnel: [w1198] -> w1193
                  tunnel: w1191 -> [w1206]
                  stop <- w1201 stop-if-true
                  n328 = Index Array(array=w1234, index #1=3 ("인덱스"), index #2=13 ("인덱스"), index #6=17 ("인덱스"), index #8=25 ("인덱스")) -> (element #1=w1203:string, element #2=w1231:string, element #3=w1226:string, element #4=w1224:string, element #5=w1215:string, element #6=w1221:string, element #7=w1220:string, element #8=w1216:string)  [unwired: 4 in]
                  n329 = Equal?(x=w1232, y=w1231) -> (x = y?=w1236:bool)
                  n330 = Equal?(x=w1237, y=w1215) -> (x = y?=w1235:bool)
                  n331 = Equal?(x=w1206, y=w1203) -> (x = y?=w1202:bool)
                  n332 = call "Unit Conversion.vi"("환산단위"=w1214, "입력단위"=w1215, "입력값"=w1231) -> ("환산값 (string)"=w1227:string)  [unwired: 3 in, 5 out]
                  n333 = call "Unit Conversion.vi"("환산단위"=w1214, "입력단위"=w1215, "입력값"=w1226) -> ("환산값 (string)"=w1225:string)  [unwired: 3 in, 5 out]
                  n334 = call "Unit Conversion.vi"("환산단위"=w1214, "입력단위"=w1215, "입력값"=w1224) -> ("환산단위"=w1223:string, "환산값 (DBL)"=w1209:dbl, "환산값 (string)"=w1200:string)  [unwired: 3 in, 3 out]
                  n335 = call "Unit Conversion.vi"("환산단위"=w1214, "입력단위"=w1220, "입력값"=w1221) -> ("환산단위"=w1218:string, "환산값 (string)"=w1219:string)  [unwired: 3 in, 4 out]
                  n336 = call "Unit Conversion.vi"("환산단위"=w1214, "입력단위"=w1215, "입력값"=w1216) -> ("환산값 (DBL)"=w1208:dbl, "환산값 (string)"=w1204:string)  [unwired: 3 in, 4 out]
                  n337 = Compound Arithmetic op=AND ("복합 연산")(w1236, w1235, w1202) -> (w1201:bool)
                  n338 = Select(t=w1234, s=w1201, f=string[] [""]) -> (s? t:f=w1230:string[])
                  n339 = Select(t=w1200, s=w1201, f="") -> (s? t:f=w1198:string)
                  n340 = Subtract(x=w1209, y=w1208) -> (x-y=w1210:dbl)
                  n341 = Absolute Value(x=w1210) -> (abs(x)=w1211:dbl)
                  n342 = Format Into String(format string="%#f" ("포맷 문자열"), w1211) -> (resulting string=w1207:string)  [unwired: 2 in, 1 out]
                  n343 = Replace Array Subset(array=w1230, new element #1=w1227, index #1=13 ("인덱스"), new element #2=w1225, new element #3=w1200, new element #4=w1223, new element #5=w1219, new element #6=w1218, new element #7=w1204, index #7=25 ("인덱스"), new element #8=w1207) -> (w1229:string[])  [unwired: 6 in]
                }
              }
            }
            n344 = Insert Into Array(array=w1187, index=1 ("인덱스"), new element=w1177) -> (w1179:string[])
          }
        }
      }
    }
    frame "Length_4" {
      w1253 = TRUE ("Write blank data ?(T)")
      n345 = call "STD Filter.vi"("Cal STD in"=w1252, "문자열(option, STD)"="Gauge Block" ("검색 문자열")) -> ("Cal STD out"=w1250:string[][], "DATA 출력"=w1251:string[][])  [unwired: 5 in, 3 out]
      n346 = call "STD Filter.vi"("Cal STD in"=w1250, "문자열(option, STD)"="Gauge Block Comparator" ("검색 문자열")) -> ("Cal STD out"=w1247:string[][], "DATA 출력"=w1249:string[][])  [unwired: 5 in, 3 out]
      n347 = call "STD Filter.vi"("Cal STD in"=w1247, "STD select"=Cmd_STD_select."Thermo-Hygrometer") -> ("DATA 출력"=w1246:string[][])  [unwired: 5 in, 4 out]
      n348 = for {
        tunnel: w1257 -> [w1260] mode=indexing
        tunnel: w1251 -> [w1262]
        tunnel: [w1259] -> w1256 mode=indexing
        n349 = Index Array(array=w1260) -> (element #1=w1258:string, element #2=w1261:string)  [unwired: 2 in]
        n350 = case shown="기본" w1258 {
          selector: w1258 -> [w1263 _]
          tunnel: w1262 -> [w1266 _]
          tunnel: w1261 -> [w1265 _]
          tunnel: [w1264 string[] ["0", "", "", "", "", "", "", "", "", "", "", "", "", "0", "0", "0", "", "0", "", "0"] ("t")] -> w1259
          frame Default {
            n351 = for {
              tunnel: w1266 -> [w1270] mode=indexing
              tunnel: w1263 -> [w1268]
              tunnel: w1265 -> [w1275]
              tunnel: [w1267] -> w1264
              stop <- w1271 stop-if-true
              n352 = Index Array(array=w1270, index #1=13 ("인덱스")) -> (element #1=w1276:string, element #4=w1274:string)  [unwired: 3 in, 2 out]
              n353 = Equal?(x=w1268, y=w1276) -> (x = y?=w1273:bool)
              n354 = Equal?(x=w1275, y=w1274) -> (x = y?=w1272:bool)
              n355 = And(x=w1273, y=w1272) -> (x .and. y?=w1271:bool)
              n356 = Select(t=w1270, s=w1271, f=string[] [""]) -> (s? t:f=w1267:string[])
            }
          }
          frame "" {
          }
        }
      }
      n357 = call "Variables Data IO.vi"("Write blank data ?(F)"=w1253, "Select"=Cmd_Var_Data_IO."STD3", "error in"=w1244, "Data In"=w1246, "Func_ext"=w1245) -> ("error out"=w1243:errorcluster, "Func_ext Out"=w1242:string)  [unwired: 4 in, 1 out]
      n358 = call "Variables Data IO.vi"("Write blank data ?(F)"=w1253, "Select"=Cmd_Var_Data_IO."STD2", "error in"=w1243, "Data In"=w1249, "Func_ext"=w1242) -> ("error out"=w1241:errorcluster)  [unwired: 4 in, 2 out]
    }
    frame "Length_5" {
      n359 = case shown="\"10503-0\"" w1281 {
        tunnel: w1284 -> [w1536 w1546 w1558 w1561]
        tunnel: ["Standard Scale" ("기준기명") w1538 w1556 w1562] -> w1283
        tunnel: [w1536 w1546 w1558 w1561] -> w1282
        tunnel: w1280 -> [_ _ w1557 _]
        tunnel: w1279 -> [_ w1537 _ _]
        frame Default {
        }
        frame "10503-0" {
          n360 = Index Array(array=w1546, index (col)=2 ("비활성화된 인덱스 (열)")) -> (element=w1544:string[])  [unwired: 1 in]
          n361 = Build Array("Step Gauge" ("기준기명"), "Gauge Block" ("기준기명")) -> (w1542:string[])
          n362 = for {
            tunnel: w1544 -> [w1555]
            tunnel: w1542 -> [w1554] mode=indexing
            tunnel: [w1554] -> w1539 mode=indexing if=w1552
            n363 = Search 1D Array(1D array=w1555, element=w1554) -> (index of element=w1553:i32)  [unwired: 1 in]
            n364 = Greater Or Equal To 0?(x=w1553) -> (x >= 0?=w1552:bool)
          }
          n365 = Array Size(array=w1539) -> (size(s)=w1540:i32)
          n366 = case shown="기본" w1540 {
            tunnel: w1539 -> [w1548 w1551]
            tunnel: [w1547 w1550] -> w1538
            tunnel: w1537 -> [_ w1549]
            frame 1 {
              n367 = Index Array(array=w1548) -> (element=w1547:string)  [unwired: 1 in]
            }
            frame Default {
              n368 = call "User select_combobox.vi"("문자열 입력"=w1549, "배열 입력"=w1551) -> ("문자열 출력"=w1550:string)  [unwired: 9 in]
            }
          }
        }
        frame "10504-1", "10511-1" {
          n369 = case shown="\"Length_5_R5\"" w1557 {
            tunnel: ["Standard Scale" ("기준기명") "Gauge Block" ("기준기명")] -> w1556
            frame Default {
            }
            frame "Length_5_R5" {
            }
          }
        }
        frame "10233-0", "10611-0" {
          n370 = Index Array(array=w1561, index (row)=0 ("인덱스 (행)"), index (col)=2 ("비활성화된 인덱스 (열)")) -> (element=w1562:string)
        }
      }
      n371 = case shown="\"Step Gauge + Gauge Block\"" w1283 {
        selector: w1283 -> [_ _ _ w1367 w1390 w1400 _ _]
        tunnel: w1287 -> [_ w1299 w1305 w1368 w1395 w1407 w1443 w1491]
        tunnel: [w1290 w1301 w1304 w1373 w1396 w1402 w1440 w1490] -> w1288
        tunnel: w1282 -> [w1290 w1297 w1303 w1366 w1392 w1401 w1446 w1494]
        tunnel: w1281 -> [_ _ _ _ w1398 _ w1450 w1498]
        tunnel: w1280 -> [_ _ _ _ w1397 _ w1451 w1499]
        tunnel: w1285 -> [w1289 w1300 w1302 w1372 w1394 w1403 w1449 w1497]
        tunnel: [w1289 w1300 w1302 w1372 w1393 w1403 w1448 w1496] -> w1286
        frame Default {
        }
        frame "Measuring Projector" {
          w1291 = "μm" ("환산단위")
          n372 = call "STD Filter.vi"("Cal STD in"=w1297, "STD select"=Cmd_STD_select."Measuring Projector") -> ("DATA 출력"=w1296:string[][], "문자열(option, STD)"=w1295:string)  [unwired: 5 in, 3 out]
          n373 = call "Match_Linear.vi"("환산단위(보정값)"=w1291, "기준기명"=w1295, "교정(T) 보정(F)"=FALSE ("교정값(T)"), "열팽창계수(etc)"="0.000008" ("열팽창계수"), "환산단위(불확도)"=w1291, "Cal STD in"=w1296, "환산단위(교정값)"="mm" ("환산단위"), "Condition Default"=w1299) -> ("Data out"=w1301:string[][])  [unwired: 2 in, 1 out]
        }
        frame "Ring Gauge" {
          n374 = for {
            tunnel: w1305 -> [w1339] mode=indexing
            tunnel: w1303 -> [w1307]
            tunnel: [w1322] -> w1304 mode=indexing
            n375 = Index Array(array=w1339) -> (element #1=w1314:string, element #2=w1313:string)  [unwired: 2 in]
            n376 = call "Unit Conversion.vi"("소수점 자리수"=2, "환산단위"="mm", "입력단위"=w1313, "입력값"=w1314) -> ("환산값 (DBL)"=w1310:dbl)  [unwired: 2 in, 5 out]
            n377 = Format Into String(format string="%#.2f" ("포맷 문자열"), w1310) -> (resulting string=w1306:string)  [unwired: 2 in, 1 out]
            n378 = for {
              tunnel: w1307 -> [w1363] mode=indexing
              tunnel: [w1362] -> w1332
              tunnel: w1306 -> [w1357]
              stop <- w1353 stop-if-true
              n379 = Index Array(array=w1363, index #1=3 ("인덱스"), index #2=13 ("인덱스")) -> (element #1=w1354:string, element #2=w1352:string)
              n380 = Equal?(x="X-X´" ("y"), y=w1354) -> (x = y?=w1359:bool)
              n381 = Equal?(x=w1352, y=w1357) -> (x = y?=w1356:bool)
              n382 = Compound Arithmetic op=AND(w1359, w1356) -> (w1353:bool)
              n383 = Select(t=w1363, s=w1353, f=string[] []) -> (s? t:f=w1362:string[])
            }
            n384 = for {
              tunnel: w1307 -> [w1351] mode=indexing
              tunnel: [w1350] -> w1308
              tunnel: w1306 -> [w1345]
              stop <- w1341 stop-if-true
              n385 = Index Array(array=w1351, index #1=3 ("인덱스"), index #2=13 ("인덱스")) -> (element #1=w1342:string, element #2=w1340:string)
              n386 = Equal?(x="Y-Y´" ("y"), y=w1342) -> (x = y?=w1347:bool)
              n387 = Equal?(x=w1340, y=w1345) -> (x = y?=w1344:bool)
              n388 = Compound Arithmetic op=AND(w1347, w1344) -> (w1341:bool)
              n389 = Select(t=w1351, s=w1341, f=string[] []) -> (s? t:f=w1350:string[])
            }
            n390 = Index Array(array=w1308, index #1=3 ("인덱스"), index #2=15 ("인덱스")) -> (element #1=w1325:string, element #2=w1323:string)
            n391 = Index Array(array=w1332, index #1=1 ("인덱스"), index #2=13 ("인덱스"), index #3=3 ("인덱스"), index #4=15 ("인덱스"), index #6=19 ("인덱스"), index #7=21 ("인덱스"), index #8=24 ("인덱스")) -> (element #1=w1330:string, element #2=w1329:string, element #3=w1328:string, element #4=w1327:string, element #5=w1321:string, element #6=w1320:string, element #7=w1319:string, element #8=w1318:string, element #9=w1317:string, element #10=w1316:string, element #11=w1315:string)  [unwired: 4 in]
            n392 = Build Array(w1330, w1329, w1328, w1327, w1325, w1323, w1321, w1320, w1319, w1318, w1317, w1316, w1315) -> (w1322:string[])
          }
        }
        frame "Standard Scale" {
          n393 = call "STD Filter.vi"("Cal STD in"=w1366, "문자열(option, STD)"=w1367) -> ("DATA 출력"=w1365:string[][], "문자열(option, STD)"=w1364:string)  [unwired: 5 in, 3 out]
          n394 = Index Array(array=w1365, index (col)=1 ("비활성화된 인덱스 (열)")) -> (element=w1380:string[])  [unwired: 1 in]
          n395 = call-poly "Array Deduplication.vi"("배열 in"=w1380) -> ("배열 out"=w1378:string[])  [unwired: 9 in, 1 out]
          n396 = for {
            tunnel: w1378 -> [w1387] mode=indexing
            tunnel: w1365 -> [w1388]
            tunnel: [w1382] -> w1379 mode=indexing
            n397 = call-poly "Data Classification.vi"("인덱스"=1, "DATA 입력"=w1388, "검색 문자열"=w1387) -> ("DATA 출력"=w1386:string[][])  [unwired: 4 in, 4 out]
            n398 = Index Array(array=w1386, index (col)=13 ("비활성화된 인덱스 (열)")) -> (element=w1384:string[])  [unwired: 1 in]
            n399 = Fract/Exp String To Number(string=w1384) -> (number=w1383:dbl[])  [unwired: 3 in, 1 out]
            n400 = Array Max & Min(array=w1383) -> (max value=w1382:dbl)  [unwired: 3 out]
          }
          n401 = Array Max & Min(array=w1379) -> (max index (indices)=w1377:i32)  [unwired: 3 out]
          n402 = Index Array(array=w1378, index=w1377) -> (element=w1376:string)
          n403 = call-poly "Data Classification.vi"("인덱스"=1, "DATA 입력"=w1365, "검색 문자열"=w1376) -> ("DATA 출력"=w1370:string[][])  [unwired: 4 in, 4 out]
          n404 = call "Match_Linear.vi"("기준기명"=w1364, "열팽창계수(etc)"="0.000008" ("열팽창계수"), "환산단위(불확도)"="μm" ("환산단위2"), "Cal STD in"=w1370, "환산단위(교정값)"="mm" ("환산단위1"), "Condition Default"=w1368) -> ("Data out"=w1373:string[][])  [unwired: 4 in, 1 out]
        }
        frame "Gauge Block" {
          n405 = call "STD Filter.vi"("Cal STD in"=w1392, "문자열(option, STD)"=w1390) -> ("DATA 출력"=w1391:string[][])  [unwired: 5 in, 4 out]
          n406 = call "Match_Gauge Block.vi"("Calibration Default"=w1395, "세부분류코드"=w1398, "Cal STD"=w1391, "에러 입력"=w1394, "Func_ext in"=w1397) -> ("에러 출력"=w1393:errorcluster, "CalSTD"=w1396:string[][])  [unwired: 3 in, 2 out]
        }
        frame "Step Gauge" {
          n407 = Index Array(array=w1407, index (col) #1=0 ("비활성화된 인덱스 (열)")) -> (element #1=w1405:string[], element #2=w1404:string[])  [unwired: 3 in]
          n408 = call "STD Filter.vi"("Cal STD in"=w1401, "문자열(option, STD)"=w1400) -> ("DATA 출력"=w1399:string[][])  [unwired: 5 in, 4 out]
          n409 = for {
            tunnel: w1405 -> [w1410] mode=indexing
            tunnel: w1404 -> [w1413] mode=indexing
            tunnel: "mm" ("환산단위") -> [w1414]
            tunnel: [w1412] -> w1402 mode=indexing
            tunnel: w1399 -> [w1411]
            n410 = call "Unit Conversion.vi"("환산단위"=w1414, "입력단위"=w1413, "입력값"=w1410) -> ("환산값 (string)"=w1409:string)  [unwired: 3 in, 5 out]
            n411 = for {
              tunnel: w1411 -> [w1418] mode=indexing
              tunnel: w1409 -> [w1415]
              tunnel: [w1417] -> w1412 if=w1416
              stop <- w1416 stop-if-true
              n412 = case shown="기본" w1415 {
                selector: w1415 -> [w1431 _]
                tunnel: [w1435 TRUE] -> w1416
                tunnel: w1418 -> [w1434 _]
                tunnel: [w1429 string[] ["Zero", "0"]] -> w1417
                frame Default {
                  n413 = Index Array(array=w1434, index #1=2 ("인덱스"), index #2=13 ("인덱스"), index #3=15 ("인덱스"), index #5=19 ("인덱스")) -> (element #1=w1427:string, element #2=w1430:string, element #3=w1426:string, element #4=w1422:string, element #5=w1421:string, element #6=w1425:string, element #7=w1424:string, element #8=w1423:string, element #9=w1420:string, element #10=w1419:string)  [unwired: 6 in]
                  n414 = Equal?(x=w1431, y=w1430) -> (x = y?=w1435:bool)
                  n415 = Build Array(w1427, w1430, w1422, w1426, w1422, w1421, w1425, w1424, w1423, w1420, w1419) -> (w1429:string[])
                }
                frame "0" {
                }
              }
            }
          }
        }
        frame "Step Gauge + Gauge Block" {
          n416 = call "STD Filter.vi"("Cal STD in"=w1446, "문자열(option, STD)"="Gauge Block" ("기준기명")) -> ("DATA 출력"=w1444:string[][])  [unwired: 5 in, 4 out]
          n417 = call "STD Filter.vi"("Cal STD in"=w1446, "문자열(option, STD)"="Step Gauge" ("기준기명")) -> ("DATA 출력"=w1452:string[][])  [unwired: 5 in, 4 out]
          n418 = call "Match_Gauge Block.vi"("Calibration Default"=w1443, "세부분류코드"=w1450, "Cal STD"=w1444, "에러 입력"=w1449, "Func_ext in"=w1451) -> ("에러 출력"=w1448:errorcluster, "CalSTD"=w1441:string[][])  [unwired: 3 in, 2 out]
          n419 = Index Array(array=w1443, index (col) #1=0 ("비활성화된 인덱스 (열)")) -> (element #1=w1454:string[], element #2=w1453:string[])  [unwired: 3 in]
          n420 = for {
            tunnel: w1454 -> [w1458] mode=indexing
            tunnel: w1453 -> [w1461] mode=indexing
            tunnel: "mm" ("환산단위") -> [w1462]
            tunnel: [w1460] -> w1442 mode=indexing
            tunnel: w1452 -> [w1459]
            n421 = call "Unit Conversion.vi"("환산단위"=w1462, "입력단위"=w1461, "입력값"=w1458) -> ("환산값 (string)"=w1457:string)  [unwired: 3 in, 5 out]
            n422 = for {
              tunnel: w1459 -> [w1466] mode=indexing
              tunnel: w1457 -> [w1463]
              tunnel: [w1465] -> w1460 if=w1464
              stop <- w1464 stop-if-true
              n423 = case shown="기본" w1463 {
                selector: w1463 -> [w1479 _]
                tunnel: [w1483 TRUE] -> w1464
                tunnel: w1466 -> [w1482 _]
                tunnel: [w1477 string[] ["Zero", "0"]] -> w1465
                frame Default {
                  n424 = Index Array(array=w1482, index #1=2 ("인덱스"), index #2=13 ("인덱스"), index #3=15 ("인덱스"), index #5=19 ("인덱스")) -> (element #1=w1475:string, element #2=w1478:string, element #3=w1474:string, element #4=w1470:string, element #5=w1469:string, element #6=w1473:string, element #7=w1472:string, element #8=w1471:string, element #9=w1468:string, element #10=w1467:string)  [unwired: 6 in]
                  n425 = Equal?(x=w1479, y=w1478) -> (x = y?=w1483:bool)
                  n426 = Build Array(w1475, w1478, w1470, w1474, w1470, w1469, w1473, w1472, w1471, w1468, w1467) -> (w1477:string[])
                }
                frame "0" {
                }
              }
            }
          }
          n427 = Build Array(w1442, w1441) -> (w1439:string[][][])
          n428 = call "Match_Cal STD.vi"("Condition Default"=w1443, "Data in"=w1439, "Cal STD"=w1439) -> ("Cal STD"=w1440:string[][])  [unwired: 6 in, 2 out]
        }
        frame "Gauge Block + Step Gauge" {
          n429 = call "STD Filter.vi"("Cal STD in"=w1494, "문자열(option, STD)"="Gauge Block" ("기준기명")) -> ("DATA 출력"=w1492:string[][])  [unwired: 5 in, 4 out]
          n430 = call "STD Filter.vi"("Cal STD in"=w1494, "문자열(option, STD)"="Step Gauge" ("기준기명")) -> ("DATA 출력"=w1500:string[][])  [unwired: 5 in, 4 out]
          n431 = call "Match_Gauge Block.vi"("Calibration Default"=w1491, "세부분류코드"=w1498, "Cal STD"=w1492, "에러 입력"=w1497, "Func_ext in"=w1499) -> ("에러 출력"=w1496:errorcluster, "CalSTD"=w1489:string[][])  [unwired: 3 in, 2 out]
          n432 = Index Array(array=w1491, index (col) #1=0 ("비활성화된 인덱스 (열)")) -> (element #1=w1502:string[], element #2=w1501:string[])  [unwired: 3 in]
          n433 = for {
            tunnel: w1502 -> [w1506] mode=indexing
            tunnel: w1501 -> [w1509] mode=indexing
            tunnel: "mm" ("환산단위") -> [w1510]
            tunnel: [w1508] -> w1488 mode=indexing
            tunnel: w1500 -> [w1507]
            n434 = call "Unit Conversion.vi"("환산단위"=w1510, "입력단위"=w1509, "입력값"=w1506) -> ("환산값 (string)"=w1505:string)  [unwired: 3 in, 5 out]
            n435 = for {
              tunnel: w1507 -> [w1514] mode=indexing
              tunnel: w1505 -> [w1511]
              tunnel: [w1513] -> w1508 if=w1512
              stop <- w1512 stop-if-true
              n436 = case shown="기본" w1511 {
                selector: w1511 -> [w1527 _]
                tunnel: [w1531 TRUE] -> w1512
                tunnel: w1514 -> [w1530 _]
                tunnel: [w1525 string[] ["Zero", "0"]] -> w1513
                frame Default {
                  n437 = Index Array(array=w1530, index #1=2 ("인덱스"), index #2=13 ("인덱스"), index #3=15 ("인덱스"), index #5=19 ("인덱스")) -> (element #1=w1523:string, element #2=w1526:string, element #3=w1522:string, element #4=w1518:string, element #5=w1517:string, element #6=w1521:string, element #7=w1520:string, element #8=w1519:string, element #9=w1516:string, element #10=w1515:string)  [unwired: 6 in]
                  n438 = Equal?(x=w1527, y=w1526) -> (x = y?=w1531:bool)
                  n439 = Build Array(w1523, w1526, w1518, w1522, w1518, w1517, w1521, w1520, w1519, w1516, w1515) -> (w1525:string[])
                }
                frame "0" {
                }
              }
            }
          }
          n440 = Build Array(w1489, w1488) -> (w1487:string[][][])
          n441 = call "Match_Cal STD.vi"("Condition Default"=w1491, "Data in"=w1487, "Cal STD"=w1487) -> ("Cal STD"=w1490:string[][])  [unwired: 6 in, 2 out]
        }
      }
    }
    frame "Length_6_1" {
      w1565 = "μm" ("환산단위")
      n442 = call "STD Filter.vi"("Cal STD in"=w1571, "문자열(option, STD)"="Standard Optical Flat" ("검색 문자열")) -> ("Cal STD out"=w1568:string[][], "DATA 출력"=w1569:string[][])  [unwired: 5 in, 3 out]
      n443 = for {
        tunnel: w1573 -> [w1620] mode=indexing
        tunnel: [w1608] -> w1572 mode=indexing
        i -> [w1619]
        n444 = Index Array(array=w1620) -> (element #1=w1615:string, element #2=w1614:string)  [unwired: 2 in]
        n445 = Format Into String(format string="%s %s" ("포맷 문자열"), w1615, w1614) -> (resulting string=w1612:string)  [unwired: 2 in, 1 out]
        n446 = To Double Precision Float(number=w1619) -> (double precision float=w1617:dbl)
        n447 = Build Array(w1612) -> (w1610:string[])
        n448 = Quotient & Remainder(x=w1617, y=2.0) -> (x-y*floor(x/y)=w1616:dbl)  [unwired: 1 out]
        n449 = Equal To 0?(x=w1616) -> (x = 0?=w1611:bool)
        n450 = Select(t=w1610, s=w1611, f=string[] []) -> (s? t:f=w1608:string[])
      }
      n451 = call "STD Filter.vi"("Cal STD in"=w1568, "문자열(option, STD)"="Monochromatic Light Source" ("검색 문자열")) -> ("DATA 출력"=w1566:string[][])  [unwired: 5 in, 4 out]
      n452 = Index Array(array=w1569) -> (element=w1591:string[])  [unwired: 2 in]
      n453 = Index Array(array=w1566) -> (element=w1589:string[])  [unwired: 2 in]
      n454 = Index Array(array=w1591, index #1=1 ("인덱스"), index #3=15 ("인덱스"), index #5=19 ("인덱스")) -> (element #1=w1604:string, element #2=w1603:string, element #3=w1601:string, element #4=w1600:string, element #5=w1596:string, element #7=w1595:string, element #8=w1592:string)  [unwired: 5 in, 1 out]
      n455 = Index Array(array=w1589, index #1=1 ("인덱스"), index #3=15 ("인덱스"), index #5=19 ("인덱스")) -> (element #1=w1576:string, element #2=w1577:string, element #3=w1579:string, element #4=w1580:string, element #5=w1584:string, element #7=w1585:string, element #8=w1588:string)  [unwired: 5 in, 1 out]
      n456 = call "Unit Conversion.vi"("환산단위"=w1565, "입력단위"=w1600, "입력값"=w1601) -> ("환산단위"=w1598:string, "환산값 (string)"=w1599:string)  [unwired: 3 in, 4 out]
      n457 = call "Unit Conversion.vi"("환산단위"=w1565, "입력단위"=w1595, "입력값"=w1596) -> ("환산단위"=w1593:string, "환산값 (string)"=w1594:string)  [unwired: 3 in, 4 out]
      n458 = call "Unit Conversion.vi"("환산단위"=w1565, "입력단위"=w1580, "입력값"=w1579) -> ("환산단위"=w1582:string, "환산값 (string)"=w1581:string)  [unwired: 3 in, 4 out]
      n459 = call "Unit Conversion.vi"("환산단위"=w1565, "입력단위"=w1585, "입력값"=w1584) -> ("환산단위"=w1587:string, "환산값 (string)"=w1586:string)  [unwired: 3 in, 4 out]
      n460 = Build Array(w1604, w1603, w1599, w1598, w1594, w1593, w1592) -> (w1606:string[])
      n461 = Build Array(w1576, w1577, w1581, w1582, w1586, w1587, w1588) -> (w1574:string[])
      n462 = Build Array(w1606, w1574) -> (w1590:string[][])
    }
    frame "Length_6_2" {
      n463 = call "STD Filter.vi"("Cal STD in"=w1623, "문자열(option, STD)"="Gauge Block Comparator" ("검색 문자열")) -> ("DATA 출력"=w1622:string[][])  [unwired: 5 in, 4 out]
      n464 = for {
        tunnel: [w1653] -> w1626 mode=indexing
        tunnel: w1622 -> [w1643] mode=indexing
        w1632 = "μm" ("환산단위")
        n465 = Index Array(array=w1643, index #1=1 ("인덱스"), index #4=15 ("인덱스"), index #8=19 ("인덱스")) -> (element #1=w1634:string, element #2=w1652:string, element #3=w1651:string, element #4=w1649:string, element #5=w1648:string, element #6=w1638:string, element #7=w1637:string, element #8=w1639:string, element #10=w1641:string, element #11=w1642:string)  [unwired: 8 in, 1 out]
        n466 = call "Unit Conversion.vi"("환산단위"=w1632, "입력단위"=w1648, "입력값"=w1649) -> ("환산단위"=w1646:string, "환산값 (string)"=w1647:string)  [unwired: 3 in, 4 out]
        n467 = call "Unit Conversion.vi"("환산단위"=w1632, "입력단위"=w1637, "입력값"=w1638) -> ("환산단위"=w1635:string, "환산값 (string)"=w1636:string)  [unwired: 3 in, 4 out]
        n468 = call "Unit Conversion.vi"("환산단위"=w1632, "입력단위"=w1641, "입력값"=w1639) -> ("환산단위"=w1644:string, "환산값 (string)"=w1645:string)  [unwired: 3 in, 4 out]
        n469 = Build Array(w1634, w1652, w1651, w1647, w1646, w1636, w1635, w1645, w1644, w1642) -> (w1653:string[])
      }
      n470 = for {
        tunnel: w1625 -> [_] mode=indexing
        tunnel: [w1629] -> w1621 mode=indexing
        w1630 = "0.01" ("원소")
        n471 = Build Array("Digital" ("원소"), w1630, w1630, "μm" ("환산단위")) -> (w1629:string[])
      }
    }
    frame "Length_7" {
      n472 = case shown="기본" w1660 {
        selector: w1660 -> [_ w1713 w1738 w1760 w1765]
        tunnel: w1663 -> [w1672 w1716 w1733 w1755 w1768]
        tunnel: [w1671 w1719 w1737 w1759 w1772] -> w1662
        tunnel: w1661 -> [w1667 w1705 w1731 w1753 w1767]
        tunnel: [w1669 w1718 w1736 w1758 w1771] -> w1659
        tunnel: [string[] ["기준기명", "보정값"] w1717 w1735 w1757 w1770] -> w1658
        tunnel: w1657 -> [w1670 w1711 w1724 w1746 w1769]
        tunnel: [w1670 w1708 w1734 w1756 w1766] -> w1656
        tunnel: w1655 -> [_ w1712 w1725 w1747 w1764]
        tunnel: w1654 -> [_ _ w1730 w1752 _]
        frame Default {
          n473 = call "STD Filter.vi"("Cal STD in"=w1667, "문자열(option, STD)"="Standard Measuring Machine" ("검색 문자열")) -> ("DATA 출력"=w1666:string[][], "문자열(option, STD)"=w1664:string)  [unwired: 5 in, 3 out]
          n474 = for {
            tunnel: w1666 -> [w1704]
            tunnel: w1672 -> [w1692] mode=indexing
            tunnel: [w1701] -> w1671 mode=indexing
            tunnel: [w1674] -> w1669 mode=indexing
            tunnel: w1664 -> [w1675]
            w1680 = 0 ("인덱스 (열)")
            n475 = Index Array(array=w1692) -> (element #1=w1682:string, element #2=w1681:string)  [unwired: 2 in]
            n476 = Index Array(array=w1704, index (row) #1=w1680, index (col) #1=16 ("비활성화된 인덱스 (열)"), index (row) #2=w1680, index (col) #2=1 ("비활성화된 인덱스 (열)"), index (col) #3=13 ("인덱스 (행)"), index (col) #4=17 ("인덱스 (행)"), index (row) #5=w1680, index (col) #5=18 ("인덱스 (행)")) -> (element #1=w1676:string, element #2=w1677:string, element #3=w1688:string[], element #4=w1686:string[], element #5=w1684:string, element #6=w1698:string, element #7=w1690:string, element #8=w1691:string, element #9=w1683:string)  [unwired: 10 in]
            n477 = call "Unit Conversion.vi"("환산단위"=w1676, "입력단위"=w1681, "입력값"=w1682) -> ("환산값 (DBL)"=w1696:dbl)  [unwired: 3 in, 5 out]
            n478 = call "Unit Conversion.vi"("환산단위"="μm", "입력단위"=w1691, "입력값"=w1698) -> ("환산단위"=w1693:string, "환산값 (string)"=w1694:string)  [unwired: 3 in, 4 out]
            n479 = Fract/Exp String To Number(string=w1688) -> (number=w1700:dbl[])  [unwired: 3 in, 1 out]
            n480 = Fract/Exp String To Number(string=w1686) -> (number=w1703:dbl[])  [unwired: 3 in, 1 out]
            n481 = Threshold 1D Array(2:w1696, 3:w1700) -> (0:w1697:dbl)  [unwired: 1 in]
            n482 = Interpolate 1D Array(1:w1697, 2:w1703) -> (0:w1702:dbl)
            n483 = Format Into String(format string="%#.2g" ("포맷 문자열"), w1702) -> (resulting string=w1673:string)  [unwired: 2 in, 1 out]
            n484 = Build Array(w1675, w1673) -> (w1674:string[])
            n485 = Build Array(w1677, w1682, w1681, w1673, w1684, w1694, w1690, w1693, w1683) -> (w1701:string[])
          }
        }
        frame "10235-2" {
          n486 = call "STD Filter.vi"("Cal STD in"=w1705, "문자열(option, STD)"="Surface Plate" ("검색 문자열")) -> ("DATA 출력"=w1706:string[][])  [unwired: 5 in, 4 out]
          n487 = call "Variables Data IO.vi"("Write blank data ?(F)"=TRUE ("Write blank data ?(T)"), "Select"=Cmd_Var_Data_IO."STD2", "error in"=w1711, "Data In"=w1706, "Func_ext"=w1712) -> ("error out"=w1709:errorcluster, "Func_ext Out"=w1710:string)  [unwired: 4 in, 1 out]
          n488 = call "Match_Gauge Block.vi"("Calibration Default"=w1716, "세부분류코드"=w1713, "Cal STD"=w1705, "에러 입력"=w1709, "Func_ext in"=w1710) -> ("에러 출력"=w1708:errorcluster, "Data Out 2"=w1717:string[], "Data Out"=w1718:string[][], "CalSTD"=w1719:string[][])  [unwired: 3 in]
        }
        frame "10224-1", "10232-1" {
          w1739 = TRUE ("Write blank data ?(T)")
          n489 = call "STD Filter.vi"("Cal STD in"=w1731, "STD select"=Cmd_STD_select."Electronic Micrometer", "문자열(option, STD)"=w1730) -> ("Cal STD out"=w1727:string[][], "DATA 출력"=w1729:string[][])  [unwired: 4 in, 3 out]
          n490 = call "STD Filter.vi"("Cal STD in"=w1727, "문자열(option, STD)"="Surface Plate" ("검색 문자열")) -> ("DATA 출력"=w1726:string[][])  [unwired: 5 in, 4 out]
          n491 = call "Variables Data IO.vi"("Write blank data ?(F)"=w1739, "Select"=Cmd_Var_Data_IO."STD3", "error in"=w1724, "Data In"=w1726, "Func_ext"=w1725) -> ("error out"=w1722:errorcluster, "Func_ext Out"=w1723:string)  [unwired: 4 in, 1 out]
          n492 = call "Variables Data IO.vi"("Write blank data ?(F)"=w1739, "Select"=Cmd_Var_Data_IO."STD2", "error in"=w1722, "Data In"=w1729, "Func_ext"=w1723) -> ("error out"=w1721:errorcluster, "Func_ext Out"=w1720:string)  [unwired: 4 in, 1 out]
          n493 = call "Match_Gauge Block.vi"("Calibration Default"=w1733, "세부분류코드"=w1738, "Cal STD"=w1731, "에러 입력"=w1721, "Func_ext in"=w1720) -> ("에러 출력"=w1734:errorcluster, "Data Out 2"=w1735:string[], "Data Out"=w1736:string[][], "CalSTD"=w1737:string[][])  [unwired: 3 in]
        }
        frame "10232-2" {
          w1761 = TRUE ("Write blank data ?(T)")
          n494 = call "STD Filter.vi"("Cal STD in"=w1753, "STD select"=Cmd_STD_select."Electronic Micrometer", "문자열(option, STD)"=w1752) -> ("Cal STD out"=w1749:string[][], "DATA 출력"=w1751:string[][])  [unwired: 4 in, 3 out]
          n495 = call "STD Filter.vi"("Cal STD in"=w1749, "문자열(option, STD)"="Surface Plate" ("검색 문자열")) -> ("DATA 출력"=w1748:string[][])  [unwired: 5 in, 4 out]
          n496 = call "Variables Data IO.vi"("Write blank data ?(F)"=w1761, "Select"=Cmd_Var_Data_IO."STD3", "error in"=w1746, "Data In"=w1748, "Func_ext"=w1747) -> ("error out"=w1744:errorcluster, "Func_ext Out"=w1745:string)  [unwired: 4 in, 1 out]
          n497 = call "Variables Data IO.vi"("Write blank data ?(F)"=w1761, "Select"=Cmd_Var_Data_IO."STD2", "error in"=w1744, "Data In"=w1751, "Func_ext"=w1745) -> ("error out"=w1743:errorcluster, "Func_ext Out"=w1742:string)  [unwired: 4 in, 1 out]
          n498 = call "Match_Gauge Block.vi"("Calibration Default"=w1755, "세부분류코드"=w1760, "Cal STD"=w1753, "에러 입력"=w1743, "Func_ext in"=w1742) -> ("에러 출력"=w1756:errorcluster, "Data Out 2"=w1757:string[], "Data Out"=w1758:string[][], "CalSTD"=w1759:string[][])  [unwired: 3 in]
        }
        frame "10209-0" {
          n499 = call "Match_Gauge Block.vi"("Calibration Default"=w1768, "세부분류코드"=w1765, "Cal STD"=w1767, "에러 입력"=w1769, "Func_ext in"=w1764) -> ("에러 출력"=w1766:errorcluster, "Data Out 2"=w1770:string[], "Data Out"=w1771:string[][], "CalSTD"=w1772:string[][])  [unwired: 3 in]
        }
      }
    }
    frame "Length_8" {
      n500 = call "STD Filter.vi"("Cal STD in"=w1782, "STD select"=Cmd_STD_select."Electronic Micrometer", "문자열(option, STD)"=w1783) -> ("DATA 출력"=w1775:string[][])  [unwired: 4 in, 4 out]
      n501 = call "Variables Data IO.vi"("Write blank data ?(F)"=TRUE ("Write blank data ?(T)"), "Select"=Cmd_Var_Data_IO."STD2", "error in"=w1788, "Data In"=w1775, "Func_ext"=w1779) -> ("Func_ext Out"=w1774:string)  [unwired: 4 in, 2 out]
      n502 = case shown="\"10224-1\"" w1778 {
        selector: w1778 -> [w1797 w1807]
        tunnel: w1788 -> [w1795 w1805]
        tunnel: [w1800 w1811] -> w1787
        tunnel: w1786 -> [w1801 w1812]
        tunnel: [w1798 w1809] -> w1785
        tunnel: w1784 -> [_ w1804]
        tunnel: w1782 -> [w1790 w1806]
        tunnel: [w1799 w1810] -> w1781
        tunnel: [w1793 w1808] -> w1780
        tunnel: w1774 -> [w1796 _]
        frame "10224-1" {
          n503 = call "STD Filter.vi"("Cal STD in"=w1790, "문자열(option, STD)"="Surface Plate" ("검색 문자열")) -> ("DATA 출력"=w1791:string[][])  [unwired: 5 in, 4 out]
          n504 = call "Variables Data IO.vi"("Write blank data ?(F)"=TRUE ("Write blank data ?(T)"), "Select"=Cmd_Var_Data_IO."STD3", "error in"=w1795, "Data In"=w1791, "Func_ext"=w1796) -> ("error out"=w1794:errorcluster, "Func_ext Out"=w1792:string)  [unwired: 4 in, 1 out]
          n505 = call "Match_Gauge Block.vi"("Calibration Default"=w1801, "세부분류코드"=w1797, "Cal STD"=w1790, "에러 입력"=w1794, "Func_ext in"=w1792) -> ("에러 출력"=w1793:errorcluster, "Data Out 2"=w1798:string[], "Data Out"=w1799:string[][], "CalSTD"=w1800:string[][])  [unwired: 3 in]
        }
        frame Default {
          # "10206-0, 10610-0"
          n506 = call "Match_Gauge Block.vi"("Data in"=w1804, "Calibration Default"=w1812, "세부분류코드"=w1807, "Cal STD"=w1806, "에러 입력"=w1805) -> ("에러 출력"=w1808:errorcluster, "Data Out 2"=w1809:string[], "Data Out"=w1810:string[][], "CalSTD"=w1811:string[][])  [unwired: 3 in]
        }
      }
    }
    frame "Length_9" {
      n507 = call "STD Filter.vi"("Cal STD in"=w1815, "STD select"=Cmd_STD_select."Measuring Projector") -> ("제외 DATA 출력"=w1813:string[][], "DATA 출력"=w1814:string[][])  [unwired: 5 in, 3 out]
      n508 = for {
        tunnel: w1814 -> [w1853]
        tunnel: w1818 -> [w1860] mode=indexing
        tunnel: [w1863] -> w1819 mode=indexing
        tunnel: w1813 -> [w1851]
        tunnel: [w1835] -> w1817 mode=indexing
        w1825 = 0 ("인덱스 (열)")
        n509 = Index Array(array=w1860) -> (element #1=w1846:string, element #2=w1847:string, element #5=w1821:string, element #6=w1822:string)  [unwired: 6 in, 2 out]
        n510 = Equal?(x=w1847, y="가로방향") -> (x = y?=w1852:bool)
        n511 = Select(t=w1853, s=w1852, f=w1851) -> (s? t:f=w1850:string[][])
        n512 = Equal?(x=w1846, y="선재지름") -> (x = y?=w1839:bool)
        n513 = Index Array(array=w1850, index (row) #1=w1825, index (col) #1=1 ("비활성화된 인덱스 (열)"), index (col) #2=13 ("인덱스 (행)"), index (col) #3=17 ("인덱스 (행)"), index (row) #4=w1825, index (col) #4=19 ("인덱스 (행)"), index (row) #8=w1825, index (col) #8=24 ("비활성화된 인덱스 (열)")) -> (element #1=w1848:string, element #2=w1858:string[], element #3=w1856:string[], element #4=w1830:string, element #5=w1829:string, element #6=w1828:string, element #7=w1827:string, element #8=w1824:string)  [unwired: 8 in]
        n514 = Select(t="Wire" ("y"), s=w1839, f="Opening" ("y")) -> (s? t:f=w1836:string)
        n515 = Fract/Exp String To Number(string=w1821) -> (number=w1832:dbl)  [unwired: 3 in, 1 out]
        n516 = Fract/Exp String To Number(string=w1858) -> (number=w1844:dbl[])  [unwired: 3 in, 1 out]
        n517 = Fract/Exp String To Number(string=w1856) -> (number=w1864:dbl[])  [unwired: 3 in, 1 out]
        n518 = Build Array(w1836, w1821, w1822) -> (w1835:string[])
        n519 = Array Max & Min(array=w1844) -> (max value=w1843:dbl, min value=w1842:dbl)  [unwired: 2 out]
        n520 = In Range and Coerce(upper limit=w1843, x=w1832, lower limit=w1842) -> (coerced(x)=w1840:dbl, In Range?=w1841:bool)
        n521 = call "Unit Conversion.vi"("환산단위"="μm", "입력단위"=w1828, "입력값"=w1830) -> ("환산단위"=w1823:string, "환산값 (string)"=w1861:string)  [unwired: 3 in, 4 out]
        n522 = case shown="참" w1841 {
          tunnel: w1864 -> [_ w1872]
          tunnel: ["기준기범위초과" w1870] -> w1834
          tunnel: w1844 -> [_ w1867]
          tunnel: w1840 -> [_ w1866]
          frame False {
          }
          frame True {
            n523 = Threshold 1D Array(2:w1866, 3:w1867) -> (0:w1869:dbl)  [unwired: 1 in]
            n524 = Interpolate 1D Array(1:w1869, 2:w1872) -> (0:w1871:dbl)
            n525 = Format Into String(format string="%#g" ("포맷 문자열"), w1871) -> (resulting string=w1870:string)  [unwired: 2 in, 1 out]
          }
        }
        n526 = call "Unit Conversion.vi"("환산단위"=w1822, "입력단위"=w1823, "입력값"=w1834) -> ("환산단위"=w1831:string, "환산값 (string)"=w1833:string)  [unwired: 3 in, 4 out]
        n527 = Build Array(w1848, w1821, w1822, w1833, w1831, w1861, w1829, w1823, w1827, w1824) -> (w1863:string[])
      }
    }
    frame "Magnification_1" {
      n528 = call "STD Filter.vi"("Cal STD in"=w1876, "문자열(option, STD)"="Standard Scale" ("검색 문자열")) -> ("DATA 출력"=w1874:string[][], "문자열(option, STD)"=w1873:string)  [unwired: 5 in, 3 out]
      n529 = Index Array(array=w1874, index (col)=1 ("비활성화된 인덱스 (열)")) -> (element=w1891:string[])  [unwired: 1 in]
      n530 = call-poly "Array Deduplication.vi"("배열 in"=w1891) -> ("배열 out"=w1889:string[])  [unwired: 9 in, 1 out]
      n531 = for {
        tunnel: w1889 -> [w1898] mode=indexing
        tunnel: w1874 -> [w1899]
        tunnel: [w1893] -> w1890 mode=indexing
        n532 = call-poly "Data Classification.vi"("인덱스"=1, "DATA 입력"=w1899, "검색 문자열"=w1898) -> ("DATA 출력"=w1897:string[][])  [unwired: 4 in, 4 out]
        n533 = Index Array(array=w1897, index (col)=13 ("비활성화된 인덱스 (열)")) -> (element=w1895:string[])  [unwired: 1 in]
        n534 = Fract/Exp String To Number(string=w1895) -> (number=w1894:dbl[])  [unwired: 3 in, 1 out]
        n535 = Array Max & Min(array=w1894) -> (max value=w1893:dbl)  [unwired: 3 out]
      }
      n536 = Array Max & Min(array=w1890) -> (min index (indices)=w1881:i32)  [unwired: 3 out]
      n537 = Index Array(array=w1889, index=w1881) -> (element=w1888:string)
      n538 = call-poly "Data Classification.vi"("인덱스"=1, "DATA 입력"=w1874, "검색 문자열"=w1888) -> ("DATA 출력"=w1879:string[][])  [unwired: 4 in, 4 out]
      n539 = Index Array(array=w1879, index (col)=24 ("비활성화된 인덱스 (열)")) -> (element=w1882:string[])  [unwired: 1 in]
      n540 = call "Match_Linear.vi"("기준기명"=w1873, "열팽창계수(etc)"="0.000008" ("열팽창계수"), "환산단위(불확도)"="μm" ("환산단위2"), "Cal STD in"=w1879, "환산단위(교정값)"="mm" ("환산단위1"), "Condition Default"=w1877) -> ("Data out"=w1884:string[][])  [unwired: 4 in, 1 out]
    }
    frame "Squareness_1" {
      n541 = call "STD Filter.vi"("Cal STD in"=w1920, "STD select"=Cmd_STD_select."Precision Square") -> ("제외 DATA 출력"=w1906:string[][], "DATA 출력"=w1908:string[][], "문자열(option, STD)"=w1915:string)  [unwired: 5 in, 2 out]
      n542 = Index Array(array=w1913, index (col) #1=1 ("비활성화된 인덱스 (열)"), index (col) #3=1 ("인덱스 (열)")) -> (element #1=w1919:string[], element #2=w1918:string[], element #3=w1903:string[])  [unwired: 4 in]
      n543 = Index Array(array=w1908, index (col)=13 ("비활성화된 인덱스 (열)")) -> (element=w1910:string[])  [unwired: 1 in]
      n544 = Fract/Exp String To Number(string=w1903) -> (number=w1902:dbl[])  [unwired: 3 in, 1 out]
      n545 = Fract/Exp String To Number(string=w1910) -> (number=w1909:dbl[])  [unwired: 3 in, 1 out]
      n546 = Array Max & Min(array=w1902) -> (max value=w1901:dbl)  [unwired: 3 out]
      n547 = Array Max & Min(array=w1909) -> (max value=w1907:dbl)  [unwired: 3 out]
      n548 = Less Or Equal?(x=w1901, y=w1907) -> (x <= y?=w1912:bool)
      n549 = Select(t=w1908, s=w1912, f=w1906) -> (s? t:f=w1905:string[][])
      n550 = for {
        tunnel: w1919 -> [w1956] mode=indexing
        tunnel: w1918 -> [w1955] mode=indexing
        tunnel: [w1954] -> w1916 mode=indexing
        tunnel: w1915 -> [w1953]
        tunnel: w1905 -> [w1924]
        w1936 = "μm" ("환산단위")
        n551 = Index Array(array=w1924, index (col)=13 ("비활성화된 인덱스 (열)")) -> (element=w1926:string[])  [unwired: 1 in]
        n552 = Fract/Exp String To Number(string=w1926) -> (number=w1927:dbl[])  [unwired: 3 in, 1 out]
        n553 = Index Array(array=w1924, index (col) #1=13 ("인덱스 (행)"), index (col) #2=17 ("인덱스 (행)"), index (row) #3=0 ("인덱스 (열)"), index (col) #3=18 ("인덱스 (열)")) -> (element #1=w1945:string[], element #2=w1952:string[], element #3=w1938:string, element #4=w1935:string, element #6=w1934:string, element #7=w1931:string)  [unwired: 10 in, 1 out]
        n554 = call "Unit Conversion.vi"("환산단위"="mm", "입력단위"=w1955, "입력값"=w1956) -> ("환산단위"=w1946:string, "환산값 (DBL)"=w1923:dbl)  [unwired: 3 in, 4 out]
        n555 = Array Max & Min(array=w1927) -> (max value=w1922:dbl)  [unwired: 3 out]
        n556 = Max & Min(x=w1923, y=w1922) -> (min(x,y)=w1929:dbl)  [unwired: 1 out]
        n557 = Fract/Exp String To Number(string=w1945) -> (number=w1944:dbl[])  [unwired: 3 in, 1 out]
        n558 = Fract/Exp String To Number(string=w1952) -> (number=w1951:dbl[])  [unwired: 3 in, 1 out]
        n559 = Threshold 1D Array(2:w1929, 3:w1944) -> (0:w1942:dbl)  [unwired: 1 in]
        n560 = Interpolate 1D Array(1:w1942, 2:w1951) -> (0:w1948:dbl)
        n561 = Format Into String(format string="%#g" ("포맷 문자열"), w1929) -> (resulting string=w1928:string)  [unwired: 2 in, 1 out]
        n562 = Format Into String(format string="%#g" ("포맷 문자열"), w1948) -> (resulting string=w1939:string)  [unwired: 2 in, 1 out]
        n563 = call "Unit Conversion.vi"("환산단위"=w1936, "입력단위"=w1938, "입력값"=w1939) -> ("환산단위"=w1932:string, "환산값 (string)"=w1937:string)  [unwired: 3 in, 4 out]
        n564 = call "Unit Conversion.vi"("환산단위"=w1936, "입력단위"=w1934, "입력값"=w1935) -> ("환산값 (string)"=w1933:string)  [unwired: 3 in, 5 out]
        n565 = Build Array(w1953, w1928, w1946, w1937, w1932, w1933, w1932, w1931) -> (w1954:string[])
      }
    }
    frame "Squareness_2" {
      w1959 = TRUE ("Write blank data ?(F)")
      n566 = call "STD Filter.vi"("Cal STD in"=w1976, "STD select"=Cmd_STD_select."Electronic Micrometer", "문자열(option, STD)"=w1971) -> ("제외 DATA 출력"=w1970:string[][], "DATA 출력"=w1972:string[][])  [unwired: 4 in, 3 out]
      n567 = call "Variables Data IO.vi"("Write blank data ?(F)"=w1959, "Select"=Cmd_Var_Data_IO."STD2", "error in"=w1974, "Data In"=w1972, "Func_ext"=w1973) -> ("error out"=w1962:errorcluster, "Func_ext Out"=w1960:string)  [unwired: 4 in, 1 out]
      n568 = call "STD Filter.vi"("Cal STD in"=w1970, "문자열(option, STD)"="Surface Plate" ("검색 문자열")) -> ("제외 DATA 출력"=w1958:string[][], "DATA 출력"=w1961:string[][])  [unwired: 5 in, 3 out]
      n569 = call "Variables Data IO.vi"("Write blank data ?(F)"=w1959, "Select"=Cmd_Var_Data_IO."STD3", "error in"=w1962, "Data In"=w1961, "Func_ext"=w1960) -> ("error out"=w1969:errorcluster)  [unwired: 4 in, 2 out]
      n570 = call "STD Filter.vi"("Cal STD in"=w1958, "문자열(option, STD)"="Square Master") -> ("DATA 출력"=w1965:string[][], "문자열(option, STD)"=w1968:string)  [unwired: 5 in, 3 out]
      n571 = for {
        tunnel: [w2008] -> w1977 mode=indexing
        tunnel: w1968 -> [w2007]
        tunnel: w1965 -> [w1983]
        tunnel: w1957 -> [w1981] mode=indexing
        w1991 = "μm" ("환산단위")
        n572 = Index Array(array=w1981) -> (element #1=w1980:string, element #2=w1979:string)  [unwired: 2 in]
        n573 = Index Array(array=w1983, index (col) #1=13 ("인덱스 (행)"), index (col) #2=17 ("인덱스 (행)"), index (row) #3=0 ("인덱스 (열)"), index (col) #3=18 ("인덱스 (열)")) -> (element #1=w1978:string[], element #2=w2006:string[], element #3=w1993:string, element #4=w1990:string, element #6=w1989:string, element #7=w1986:string)  [unwired: 10 in, 1 out]
        n574 = call "Unit Conversion.vi"("환산단위"="mm", "입력단위"=w1979, "입력값"=w1980) -> ("환산단위"=w2000:string, "환산값 (DBL)"=w1982:dbl)  [unwired: 3 in, 4 out]
        n575 = Fract/Exp String To Number(string=w1978) -> (number=w1999:dbl[])  [unwired: 3 in, 1 out]
        n576 = Fract/Exp String To Number(string=w2006) -> (number=w2005:dbl[])  [unwired: 3 in, 1 out]
        n577 = Threshold 1D Array(2:w1982, 3:w1999) -> (0:w1997:dbl)  [unwired: 1 in]
        n578 = Interpolate 1D Array(1:w1997, 2:w2005) -> (0:w2002:dbl)
        n579 = Format Into String(format string="%#g" ("포맷 문자열"), w1982) -> (resulting string=w1984:string)  [unwired: 2 in, 1 out]
        n580 = Format Into String(format string="%#g" ("포맷 문자열"), w2002) -> (resulting string=w1994:string)  [unwired: 2 in, 1 out]
        n581 = call "Unit Conversion.vi"("환산단위"=w1991, "입력단위"=w1993, "입력값"=w1994) -> ("환산단위"=w1987:string, "환산값 (string)"=w1992:string)  [unwired: 3 in, 4 out]
        n582 = call "Unit Conversion.vi"("환산단위"=w1991, "입력단위"=w1989, "입력값"=w1990) -> ("환산값 (string)"=w1988:string)  [unwired: 3 in, 5 out]
        n583 = Build Array(w2007, w1984, w2000, w1992, w1987, w1988, w1987, w1986) -> (w2008:string[])
      }
    }
    frame "Flatness_1" {
      w2016 = TRUE ("Write blank data ?(F)")
      n584 = call "STD Filter.vi"("Cal STD in"=w2029, "STD select"=Cmd_STD_select."Electronic Micrometer", "문자열(option, STD)"=w2025) -> ("제외 DATA 출력"=w2024:string[][], "DATA 출력"=w2009:string[][])  [unwired: 4 in, 3 out]
      n585 = call "STD Filter.vi"("Cal STD in"=w2024, "문자열(option, STD)"="Surface Plate" ("검색 문자열")) -> ("제외 DATA 출력"=w2015:string[][], "DATA 출력"=w2010:string[][])  [unwired: 5 in, 3 out]
      n586 = call "STD Filter.vi"("Cal STD in"=w2015, "문자열(option, STD)"="Gauge Block") -> ("DATA 출력"=w2013:string[][])  [unwired: 5 in, 4 out]
      n587 = call-poly "Data Sorting.vi"("기준열"=u16 13, "Data in"=w2013) -> ("Data out"=w2012:string[][])  [unwired: 8 in, 1 out]
      n588 = for {
        tunnel: w2012 -> [w2031] mode=indexing
        tunnel: [w2031] -> w2014 mode=indexing if=w2030
        n589 = Index Array(array=w2031, index=13 ("인덱스")) -> (element=w2032:string)
        n590 = case shown="\"12\", \"13\", \"25\"" w2032 {
          tunnel: [_ TRUE] -> w2030
          frame Default {
          }
          frame "12", "13", "25" {
          }
        }
      }
      n591 = call "Variables Data IO.vi"("Write blank data ?(F)"=w2016, "Select"=Cmd_Var_Data_IO."STD3", "error in"=w2027, "Data In"=w2014, "Func_ext"=w2026) -> ("error out"=w2018:errorcluster, "Func_ext Out"=w2017:string)  [unwired: 4 in, 1 out]
      n592 = call "Variables Data IO.vi"("Write blank data ?(F)"=w2016, "Select"=Cmd_Var_Data_IO."STD2", "error in"=w2018, "Data In"=w2010, "Func_ext"=w2017) -> ("error out"=w2023:errorcluster)  [unwired: 4 in, 2 out]
    }
    frame "Straightness_1" {
      n593 = Index Array(array=w2041, index (col) #1=0 ("비활성화된 인덱스 (열)")) -> (element #1=w2040:string[], element #2=w2039:string[])  [unwired: 3 in]
      n594 = call "STD Filter.vi"("Cal STD in"=w2043, "STD select"=Cmd_STD_select."Straight Edge") -> ("DATA 출력"=w2035:string[][], "문자열(option, STD)"=w2036:string)  [unwired: 5 in, 3 out]
      n595 = for {
        tunnel: w2035 -> [w2073]
        tunnel: w2040 -> [w2067] mode=indexing
        tunnel: w2039 -> [w2066] mode=indexing
        tunnel: [w2064] -> w2037 mode=indexing
        tunnel: w2036 -> [w2054]
        w2050 = "μm" ("환산단위")
        n596 = Index Array(array=w2073, index (col) #1=13 ("인덱스 (행)"), index (col) #2=17 ("인덱스 (행)"), index (row) #3=0 ("인덱스 (열)"), index (col) #3=18 ("인덱스 (열)")) -> (element #1=w2061:string[], element #2=w2072:string[], element #3=w2052:string, element #4=w2049:string, element #6=w2048:string, element #7=w2045:string)  [unwired: 10 in, 1 out]
        n597 = call "Unit Conversion.vi"("환산단위"="mm", "입력단위"=w2066, "입력값"=w2067) -> ("환산단위"=w2062:string, "환산값 (DBL)"=w2057:dbl, "환산값 (string)"=w2063:string)  [unwired: 3 in, 3 out]
        n598 = Fract/Exp String To Number(string=w2061) -> (number=w2060:dbl[])  [unwired: 3 in, 1 out]
        n599 = Fract/Exp String To Number(string=w2072) -> (number=w2071:dbl[])  [unwired: 3 in, 1 out]
        n600 = Threshold 1D Array(2:w2057, 3:w2060) -> (0:w2058:dbl)  [unwired: 1 in]
        n601 = Interpolate 1D Array(1:w2058, 2:w2071) -> (0:w2068:dbl)
        n602 = Format Into String(format string="%#g" ("포맷 문자열"), w2068) -> (resulting string=w2053:string)  [unwired: 2 in, 1 out]
        n603 = call "Unit Conversion.vi"("환산단위"=w2050, "입력단위"=w2052, "입력값"=w2053) -> ("환산단위"=w2046:string, "환산값 (string)"=w2051:string)  [unwired: 3 in, 4 out]
        n604 = call "Unit Conversion.vi"("환산단위"=w2050, "입력단위"=w2048, "입력값"=w2049) -> ("환산값 (string)"=w2047:string)  [unwired: 3 in, 5 out]
        n605 = Build Array(w2054, w2063, w2062, w2051, w2046, w2047, w2046, w2045) -> (w2064:string[])
      }
    }
    frame Default {
      w2074 = string[][] [] ("Data out")
    }
  }
  "Cal STD" <- w23
  "Data Out" <- w28
  "Data Out 2" <- w11
  n606 = for {
    tunnel: w22 -> [w2079] mode=indexing
    tunnel: [w2076] -> w20 mode=indexing
    n607 = Concatenate Strings(w2079) -> (w2078:string)
    n608 = call <vilib>:"Trim Whitespace.vi"("string"=w2078) -> ("trimmed string"=w2077:string)  [unwired: 1 in]
    n609 = Empty String/Path?(string/path=w2077) -> (empty?=w2076:bool)
  }
  n610 = Empty Array?(array=w23) -> (empty?=w24:bool)
  "생성오류?" <- w24
  n611 = call "Variables Data IO.vi"("Write blank data ?(F)"=TRUE ("Write blank data ?(T)"), "Select"=Cmd_Var_Data_IO."STD1", "error in"=w31, "Data In"=w23, "Func_ext"="Func_ext") -> ("error out"=→"error out":errorcluster, "Func_ext Out"=→"Func_ext Out":string)  [unwired: 4 in, 1 out]
  n612 = Or Array Elements(Boolean array=w20) -> (logical OR=w19:bool)
  "데이터오류?" <- w19
  n613 = Build Array(w24, w19) -> (w14:bool[])
  n614 = global read "Global_Cal Info.vi" "Func List"() -> (w18:string[][])
  n615 = global read "Global_Cal Info.vi" "std error?"() -> (w15:bool[][])
  n616 = Index Array(array=w18, index (col)=2 ("비활성화된 인덱스 (열)")) -> (element=w17:string[])  [unwired: 1 in]
  n617 = Search 1D Array(1D array=w17, element="Func_ext") -> (index of element=w13:i32)  [unwired: 1 in]
  n618 = Replace Array Subset(array=w15, new element=w14, index (row)=w13) -> (w12:bool[][])  [unwired: 1 in]
  n619 = global write "Global_Cal Info.vi" "std error?"(w12) -> ()
